vi "vision picture 1.42.vi"() -> ()   [LabVIEW 2011]
uses:
  IMAQ Image.ctl
  <vilib>/userDefined/High Color/IMAQdx.ctl
  U16 Changed__ogtk.vi
  U32 Changed__ogtk.vi
  I32 Changed__ogtk.vi
  Variant Changed__ogtk.vi
  <vilib>/vision/driver/NI_Vision_Acquisition_Software.lvlib
panel:
  in  "Zoom":sgl=1.0 min=0.1 step=0.1 format="%#_2f"
  out "Color Image":T1={"Color Image", 228380588}
  out "Image Template Out":T1
  in  "Interface Name":u16(ring) items=["Still image", "TOSHIBA Web Camera - HD", "SplitCam Video Driver", "SplitCam Video Filter", "IP Split Camera"]
  out "Paused Original Picture":picture
  out "Paused Original Image":T1={"Paused Original Image", 212497164}
  in  "Pause":bool
  in  "Play":bool
  out "Cluster Maches Color Out":T2 {"Matches Out"."Bounding Box"."y" format="%.2f"; "Matches Out"."Bounding Box"."x" format="%.2f"; "Matches Out"."Position"."y" format="%.2f"; "Matches Out"."Position"."x" format="%.2f"; "Matches Out"."Score" format="%.2f"; "Matches Out"."Scale" format="%.2f"; "Matches Out"."Angle" format="%.2f"}
  out "Cluster Shape Report Out":T3 {"Shape Report"."Score" format="%.2f"; "Shape Report"."Centroid"."y" format="%.2f"; "Shape Report"."Centroid"."x" format="%.2f"}
  out "Cluster Particle Reports (Pixels) Out":T4 {"Particle Reports (Pixels)"."Orientation" format="%.2f"; "Particle Reports (Pixels)"."Dimensions"."Height" format="%.2f"; "Particle Reports (Pixels)"."Dimensions"."Width" format="%.2f"; "Particle Reports (Pixels)"."Center of Mass"."Y" format="%.2f"; "Particle Reports (Pixels)"."Center of Mass"."X" format="%.2f"; "Particle Reports (Pixels)"."Bounding Rect"."Bottom" format="%.2f"; "Particle Reports (Pixels)"."Bounding Rect"."Right" format="%.2f"; "Particle Reports (Pixels)"."Bounding Rect"."Top" format="%.2f"; "Particle Reports (Pixels)"."Bounding Rect"."Left" format="%.2f"; "Particle Reports (Pixels)"."Number of Holes" format="%.2f"; "Particle Reports (Pixels)"."Area" format="%.2f"}
  out "Morphology Image":T1={"Morphology Image", 205500188}
  out "Threshold Image":T1={"Threshold Image", 140289436}
  out "Rect Out":T5
  out "Result Picture":picture caption="Particle Analysis"
  out "Source Image":picture
  out "Numeric Tab control":i32
  in  "Tab Control":T6(tab)
  in  "Color Mode":u16(ring) items=["RGB", "HSL", "HSV", "HSI"]
  out "Histogram":T7(graph)
  out "BCG Image":T1={"BCGLookup Image", 211850956}
  in  "Background Correction":T8={"Brightness"=128, "Contrast"=45, "Gamma"=1.0} {"Gamma" min=0.1 max=2 step=0.01 scale=0.0..2.0; "Contrast" min=1 max=90 step=1 scale=0.0..90.0; "Brightness" min=0 max=255 step=1 scale=0.0..255.0}
  in  "Subtraction":bool
  out "Backgroud In":T1
  out "Original Image":T1={"Original Image", 139855628}
  in  "Refresh":bool
  out "High Sensitivity":dbl[][](graph)
  out "Medium Sensitivity":dbl[][](graph)
  out "Color Spectrum - Low Sensitivity":dbl[][](graph)
  in  "Saturation Threshold":i32=80 min=1 max=255 step=1
  in  "Color Sensitivity":u32(ring) caption="Color Complexity" items=["Low", "Medium", "High"]
  in  "1. Threshold":bool
  in  "3. Shape":bool
  in  "Particle Connectivity Control":bool=TRUE
  in  "4. Particle Connectivity":bool
  out "MagicWand Image":T1
  in  "Shape Control":T9={"Scale Invariance"=TRUE, "Tolerance (%)"=2.0, "Connectivity"=TRUE} {"Tolerance (%)" min=0.0 max=10.0 step=0.5 format="%.2f"}
  in  "2. Morphology":bool
  in  "Morphology Control":enum32{" 1º", " 2º", " 3º", " 4º", " 5º"}(tab)
  in  "Filter":bool
  in  "Connectivity for Particle Erosion":bool=TRUE
  in  "Neighborhood":bool
  in  "Particles to Erode":i32=2
  in  "Reject Particles Touching the Image Border":bool
  in  "Connectivity for Border Rejection":bool=TRUE
  in  "Fill Holes":bool
  in  "Connectivity for Hole Filling":bool=TRUE
  in  "Morphology for Separation Erosion":bool
  in  "Separation Erosion":i32 min=0 max=20 step=1
  out "Particles":i32
  in  "Connectivity for PF":bool=TRUE
  in  "Keep/Remove PF":bool
  in  "Particle Filter Values":T11(array[cluster]) {"Measurement Parameter" items=["Center of Mass X", "Center of Mass Y", "First Pixel X", "First Pixel Y", "Bounding Rect Left", "Bounding Rect Top", "Bounding Rect Right", "Bounding Rect Bottom", "Max Feret Diameter Start X", "Max Feret Diameter Start Y", "Max Feret Diameter End X", "Max Feret Diameter End Y", "Max Horiz. Segment Length Left", "Max Horiz. Segment Length Right", "Max Horiz. Segment Length Row", "-", "Bounding Rect Width", "Bounding Rect Height", "Bounding Rect Diagonal", "Perimeter", "Convex Hull Perimeter", "Holes' Perimeter", "Max Feret Diameter", "Equivalent Ellipse Major Axis", "Equivalent Ellipse Minor Axis", "Equivalent Ellipse Minor Axis (Feret)", "Equivalent Rect Long Side", "Equivalent Rect Short Side", "Equivalent Rect Diagonal", "Equivalent Rect Short Side (Feret)", "Average Horiz. Segment Length", "Average Vert. Segment Length", "Hydraulic Radius", "Waddel Disk Diameter", "-", "Area", "Holes' Area", "Particle & Holes' Area", "Convex Hull Area", "Image Area", "-", "Number of Holes", "Number of Horiz. Segments", "Number of Vert. Segments", "-", "Orientation", "Max Feret Diameter Orientation", "-", "% Area/Image Area", "% Area/(Particle & Holes' Area)", "Ratio of Equivalent Ellipse Axes", "Ratio of Equivalent Rect Sides", "-", "Elongation Factor", "Compactness Factor", "Heywood Circularity Factor", "Type Factor", "-", "Sum X", "Sum Y", "Sum XX", "Sum XY", "Sum YY", "Sum XXX", "Sum XXY", "Sum XYY", "Sum YYY", "-", "Moment of Inertia XX", "Moment of Inertia XY", "Moment of Inertia YY", "Moment of Inertia XXX", "Moment of Inertia XXY", "Moment of Inertia XYY", "Moment of Inertia YYY", "Norm. Moment of Inertia XX", "Norm. Moment of Inertia XY", "Norm. Moment of Inertia YY", "Norm. Moment of Inertia XXX", "Norm. Moment of Inertia XXY", "Norm. Moment of Inertia XYY", "Norm. Moment of Inertia YYY", "Hu Moment 1", "Hu Moment 2", "Hu Moment 3", "Hu Moment 4", "Hu Moment 5", "Hu Moment 6", "Hu Moment 7"]; "Lower Value Range" format="%.2f"; "Upper Value Range" format="%.2f"}
  in  "Particle Filter":bool
  in  "Threshold Control":enum32{"Automatic", "Manual"}(tab)
  in  "Color Plane":i32(ring) items=["Red", "Green", "Blue", "Hue", "Saturation", "Luminance", "Value", "Intensity"]
  out "Threshold Value":i32=77
  in  "Automatic":cluster{"Object Type":u32, "Method":i32}={"Object Type"=1, "Method"=0} {"Method" items=["clustering", "entropy", "metric", "moments", "inter-class variance"]; "Object Type" items=["Bright Objects", "Dark Objects"]}
  in  "controls threshold":T12={"Threshold Color Mode"=0, "Color Value"=1, "Cluster Color"={"Histogram Red"={"Starting Value"=0.0, "Incremental Value"=1.0, "Histogram"=[0, 0, 0, 0, 0, 0, 0, 0, 0, 0, 0, 0, 0, 0, 0, 0, 0, 0, 0, 0, 0, 0, 0, 0, 0, 0, 0, 0, 0, 0, 0, 0, 0, 0, 0, 0, 0, 0, 0, 0, 1, 12, 46, 79, 116, 20, 126, 161, 147, 65, 187, 447, 707, 298, 591, 993, 827, 185, 744, 503, 189, 105, 144, 210, 115, 21, 92, 111, 97, 14, 70, 95, 76, 6, 87, 44, 60, 17, 37, 46, 30, 20, 32, 67, 21, 30, 2, 86, 20, 23, 41, 27, 36, 2, 31, 61, 16, 15, 19, 27, 24, 10, 41, 53, 15, 3, 29, 18, 25, 0, 30, 37, 28, 11, 26, 33, 9, 31, 13, 58, 9, 16, 21, 57, 11, 26, 11, 37, 13, 25, 24, 33, 16, 12, 37, 40, 5, 10, 23, 34, 24, 1, 36, 41, 18, 32, 15, 50, 13, 31, 20, 34, 42, 6, 39, 34, 23, 38, 8, 71, 16, 30, 19, 86, 30, 22, 35, 82, 50, 22, 42, 88, 45, 43, 51, 157, 113, 3, 118, 162, 157, 14, 194, 223, 65, 142, 95, 500, 488, 153, 646, 1183, 2082, 511, 3520, 4145, 4586, 1568, 3156, 2717, 1800, 238, 463, 305, 75, 29, 17, 6, 1, 0, 0, 0, 0, 0, 0, 0, 0, 0, 0, 0, 0, 0, 0, 0, 0, 0, 0, 0, 0, 0, 0, 0, 0, 0, 0, 0, 0, 0, 0, 0, 0, 0, 0, 0, 0, 0, 0, 0, 0, 0, 0, 0, 0, 0, 0, 0]}, "Histogram Blue"={"Starting Value"=0.0, "Incremental Value"=1.0, "Histogram"=[0, 0, 0, 0, 0, 0, 0, 0, 0, 0, 0, 0, 0, 0, 0, 0, 0, 0, 0, 0, 0, 0, 0, 0, 0, 0, 0, 0, 0, 0, 0, 0, 0, 0, 0, 0, 0, 0, 0, 0, 1, 12, 46, 79, 116, 20, 126, 161, 147, 65, 187, 447, 707, 298, 591, 993, 827, 185, 744, 503, 189, 105, 144, 210, 115, 21, 92, 111, 97, 14, 70, 95, 76, 6, 87, 44, 60, 17, 37, 46, 30, 20, 32, 67, 21, 30, 2, 86, 20, 23, 41, 27, 36, 2, 31, 61, 16, 15, 19, 27, 24, 10, 41, 53, 15, 3, 29, 18, 25, 0, 30, 37, 28, 11, 26, 33, 9, 31, 13, 58, 9, 16, 21, 57, 11, 26, 11, 37, 13, 25, 24, 33, 16, 12, 37, 40, 5, 10, 23, 34, 24, 1, 36, 41, 18, 32, 15, 50, 13, 31, 20, 34, 42, 6, 39, 34, 23, 38, 8, 71, 16, 30, 19, 86, 30, 22, 35, 82, 50, 22, 42, 88, 45, 43, 51, 157, 113, 3, 118, 162, 157, 14, 194, 223, 65, 142, 95, 500, 488, 153, 646, 1183, 2082, 511, 3520, 4145, 4586, 1568, 3156, 2717, 1800, 238, 463, 305, 75, 29, 17, 6, 1, 0, 0, 0, 0, 0, 0, 0, 0, 0, 0, 0, 0, 0, 0, 0, 0, 0, 0, 0, 0, 0, 0, 0, 0, 0, 0, 0, 0, 0, 0, 0, 0, 0, 0, 0, 0, 0, 0, 0, 0, 0, 0, 0, 0, 0, 0, 0]}, "Histogram Green"={"Starting Value"=0.0, "Incremental Value"=1.0, "Histogram"=[0, 0, 0, 0, 0, 0, 0, 0, 0, 0, 0, 0, 0, 0, 0, 0, 0, 0, 0, 0, 0, 0, 0, 0, 0, 0, 0, 0, 0, 0, 0, 0, 0, 0, 0, 0, 0, 0, 0, 0, 1, 12, 46, 79, 116, 20, 126, 161, 147, 65, 187, 447, 707, 298, 591, 993, 827, 185, 744, 503, 189, 105, 144, 210, 115, 21, 92, 111, 97, 14, 70, 95, 76, 6, 87, 44, 60, 17, 37, 46, 30, 20, 32, 67, 21, 30, 2, 86, 20, 23, 41, 27, 36, 2, 31, 61, 16, 15, 19, 27, 24, 10, 41, 53, 15, 3, 29, 18, 25, 0, 30, 37, 28, 11, 26, 33, 9, 31, 13, 58, 9, 16, 21, 57, 11, 26, 11, 37, 13, 25, 24, 33, 16, 12, 37, 40, 5, 10, 23, 34, 24, 1, 36, 41, 18, 32, 15, 50, 13, 31, 20, 34, 42, 6, 39, 34, 23, 38, 8, 71, 16, 30, 19, 86, 30, 22, 35, 82, 50, 22, 42, 88, 45, 43, 51, 157, 113, 3, 118, 162, 157, 14, 194, 223, 65, 142, 95, 500, 488, 153, 646, 1183, 2082, 511, 3520, 4145, 4586, 1568, 3156, 2717, 1800, 238, 463, 305, 75, 29, 17, 6, 1, 0, 0, 0, 0, 0, 0, 0, 0, 0, 0, 0, 0, 0, 0, 0, 0, 0, 0, 0, 0, 0, 0, 0, 0, 0, 0, 0, 0, 0, 0, 0, 0, 0, 0, 0, 0, 0, 0, 0, 0, 0, 0, 0, 0, 0, 0, 0]}, "Red or Hue Range"={"Minimum Value"=0.0, "Maximum Value"=155.0}, "Green or Sat Range"={"Minimum Value"=0.0, "Maximum Value"=155.0}, "Blue or Luma or Val or Inten Range"={"Minimum Value"=0.0, "Maximum Value"=155.0}}} {"Cluster Color"."Blue or Luma or Val or Inten Range" scale=0.0..255.0; "Cluster Color"."Green or Sat Range" scale=0.0..255.0; "Cluster Color"."Red or Hue Range" scale=0.0..255.0; "Threshold Color Mode" items=["RGB", "HSL", "HSV", "HSI"]}
  out "Extract Image":T1
  in  "Pen Color":u32(colorbox)=16744448
  out "Extract Picture":picture
  in  "ROI Box":T13 {"Bottom" min=0.0; "Right" min=0.0; "Top" min=0.0; "Left" min=0.0}
  in  "Search Control":T14={"Search Strategy"=0, "Color Sensitivity"=0, "Match Feature Mode"=0, "Min Score"=700.0, "# Matches"=1, "Subpixel Accuracy"=FALSE, "Min Contrast"=10, "Match Mode"=0, "Color Score Weight"=500.0, "Rotation Range (º)"=[]} {"Rotation Range (º)"."?" format="%.2f"; "Rotation Range (º)"."?" format="%.2f"; "Color Score Weight" min=0 max=1000; "Match Mode" items=["Shift Invariant", "Rotation Invariant"]; "Match Feature Mode" items=["Color and Shape", "Color", "Shape"]; "Color Sensitivity" items=["Low Sensitivity", "Medium Sensitivity", "High Sensitivity"]; "Search Strategy" items=["Conservative", "Balance", "Aggressive", "Very Aggressive"]}
  in  "Learn Control":T15={"Saturation Threshold"=80, "Ignore Black and White "=0, "Feature Mode"=0, "Ignore Color Spectra"=[], "Learn Mode"=0} {"Learn Mode" items=["All", "Shift Information", "Rotation Information"]; "Ignore Color Spectra" format="%.2f"; "Feature Mode" items=["Color and Shape", "Color", "Shape "]; "Ignore Black and White" items=["Disabled", "Ignore Black", "Ignore White", "Ignore Black and White"]; "Saturation Threshold" min=0 max=255}
  in  "Background Subtraction":bool
  in  "Learn Template":bool
  in  "Order by":u16(ring) items=["Max. Area", "Min. Area", "Max. Center of Mass", "Min. Center of Mass", ""]
  out "Color Matching":T16 {"Particle Reports (Pixels)"."Orientation" format="%.2f"; "Particle Reports (Pixels)"."Dimensions"."Height" format="%.2f"; "Particle Reports (Pixels)"."Dimensions"."Width" format="%.2f"; "Particle Reports (Pixels)"."Center of Mass"."Y" format="%.2f"; "Particle Reports (Pixels)"."Center of Mass"."X" format="%.2f"; "Particle Reports (Pixels)"."Bounding Rect"."Bottom" format="%.2f"; "Particle Reports (Pixels)"."Bounding Rect"."Right" format="%.2f"; "Particle Reports (Pixels)"."Bounding Rect"."Top" format="%.2f"; "Particle Reports (Pixels)"."Bounding Rect"."Left" format="%.2f"; "Particle Reports (Pixels)"."Number of Holes" format="%.2f"; "Particle Reports (Pixels)"."Area" format="%.2f"}
  out "Color Matching":T17 {"Matches Out"."Bounding Box"."y" format="%.2f"; "Matches Out"."Bounding Box"."x" format="%.2f"; "Matches Out"."Position"."y" format="%.2f"; "Matches Out"."Position"."x" format="%.2f"; "Matches Out"."Score" format="%.2f"; "Matches Out"."Scale" format="%.2f"; "Matches Out"."Angle" format="%.2f"}
  in  "Order by":u16(ring) items=["Max. Score", "Min. Score", "Max. Position", "Min. Position"]
  in  "Show Results":u16(slide)
  out "Global Result":T18 {"Variance"."Ey2" format="%.2f"; "Variance"."Ex2" format="%.2f"; "Standard Deviation"."Ey" format="%.2f"; "Standard Deviation"."Ex" format="%.2f"; "Position"."Y" format="%.2f"; "Position"."X" format="%.2f"}
  in  "Order by":u16(ring) items=["Max. Object Size", "Min. Object Size", "Max. Score", "Min. Score"]
  out "Particle Analysis":T19 {"Shape Report"."Score" format="%.2f"; "Shape Report"."Centroid"."y" format="%.2f"; "Shape Report"."Centroid"."x" format="%.2f"}
  in  "Show Draw Point":T20={"Show Text"=TRUE, "Show Center"=TRUE, "Show Bounding Box"=TRUE, "Show Angle"=FALSE}
  out "stop 2":bool
  out "Acquiring":bool
  in  "stop":bool
  # "Color Histogram"
  # "Color Spectrum"
  # "Controls"
  # "If the automatic threshold does not work, try manual mode. Clear any particle with the morphology control. Click any shape to find."
  # "R/H"
  # "G/S"
  # "B/LVI"
  # "ROI"
  # "Select an object taking a square area about it on the output image. Modify the color of the ROI bounding box as desired"
  # "1. Choose the learning mode before the capturing process if wanted"
  # "2. Once learn, the searching process can be optimized"
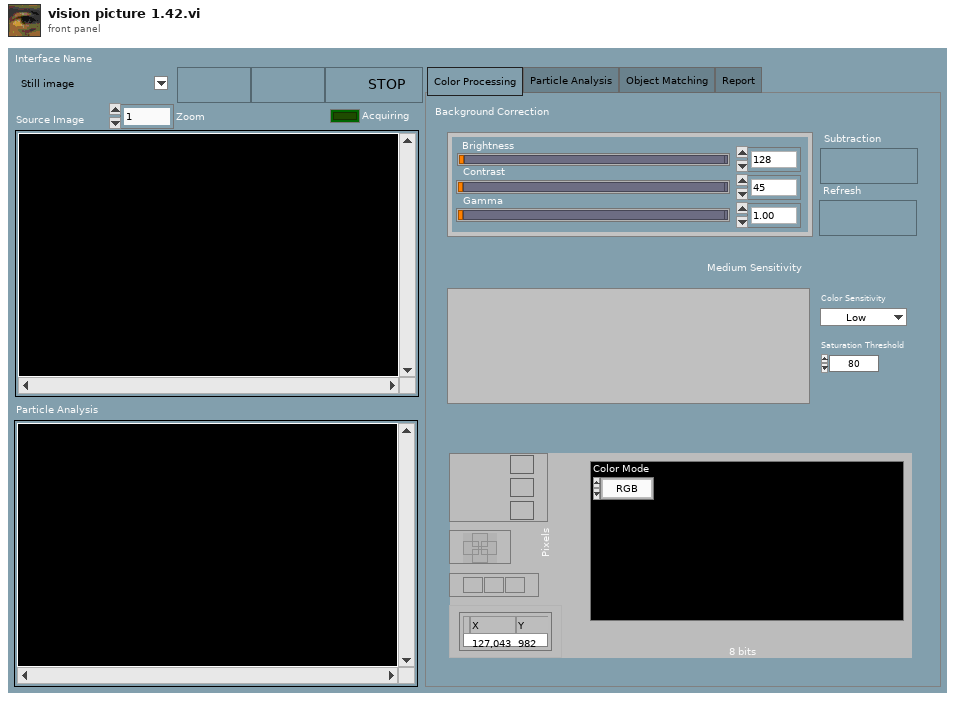
[diagram p1: front panel]
types:
  T1 = typedef "IMAQ Image.ctl" = cluster{string, u32}
  T2 = cluster{"Matches Out":cluster{"Position":cluster{"x":sgl, "y":sgl}, "Angle":sgl, "Scale":sgl, "Score":sgl, "Bounding Box":cluster{"x":sgl, "y":sgl}[]}[], "N. Matches Color":i32}
  T3 = cluster{"Shape Report":cluster{"Global Rectangle":cluster{"x1Left":i32, "y1Top":i32, "x2Right":i32, "y2Bottom":i32}, "Centroid":cluster{"x":sgl, "y":sgl}, "Object Size":u32, "Score":dbl}[], "N. Matches Shape":i32}
  T4 = cluster{"Particle Reports (Pixels)":cluster{"Area":dbl, "Number of Holes":dbl, "Bounding Rect":cluster{"Left":dbl, "Top":dbl, "Right":dbl, "Bottom":dbl}, "Center of Mass":cluster{"X":dbl, "Y":dbl}, "Orientation":dbl, "Dimensions":cluster{"Width":dbl, "Height":dbl}}[], "N. Particles Report":i32}
  T5 = cluster{"Left":i32, "Top":i32, "Right":i32, "Bottom":i32}
  T6 = enum32{"Color Processing", "Particle Analysis", "Object Matching", "Report"}
  T7 = cluster{"Starting Value":sgl, "Incremental Value":sgl, "Histogram":u32[]}[]
  T8 = cluster{"Brightness":i32, "Contrast":i32, "Gamma":sgl}
  T9 = cluster{"Scale Invariance":bool, "Tolerance (%)":dbl, "Connectivity":bool}
  T10 = typedef "Particle Parameters" = i32
  T11 = cluster{"Measurement Parameter":T10, "Lower Value Range":dbl, "Upper Value Range":dbl, "Range":bool, "Measurement Type":bool}[]
  T12 = cluster{"Threshold Color Mode":u16, "Color Value":i32, "Cluster Color":cluster{"Histogram Red":cluster{"Starting Value":sgl, "Incremental Value":sgl, "Histogram":u32[]}, "Histogram Blue":cluster{"Starting Value":sgl, "Incremental Value":sgl, "Histogram":u32[]}, "Histogram Green":cluster{"Starting Value":sgl, "Incremental Value":sgl, "Histogram":u32[]}, "Red or Hue Range":cluster{"Minimum Value":sgl, "Maximum Value":sgl}, "Green or Sat Range":cluster{"Minimum Value":sgl, "Maximum Value":sgl}, "Blue or Luma or Val or Inten Range":cluster{"Minimum Value":sgl, "Maximum Value":sgl}}}
  T13 = cluster{"Left":dbl, "Top":dbl, "Right":dbl, "Bottom":dbl}
  T14 = cluster{"Search Strategy":u32, "Color Sensitivity":u32, "Match Feature Mode":u32, "Min Score":sgl, "# Matches":i32, "Subpixel Accuracy":bool, "Min Contrast":i32, "Match Mode":u16, "Color Score Weight":sgl, "Rotation Range (º)":cluster{sgl, sgl}[]}
  T15 = cluster{"Saturation Threshold":i32, "Ignore Black and White ":u32, "Feature Mode":u32, "Ignore Color Spectra":dbl[][], "Learn Mode":u16}
  T16 = cluster{"Particle Reports (Pixels)":cluster{"Area":dbl, "Number of Holes":dbl, "Bounding Rect":cluster{"Left":dbl, "Top":dbl, "Right":dbl, "Bottom":dbl}, "Center of Mass":cluster{"X":dbl, "Y":dbl}, "Orientation":dbl, "Dimensions":cluster{"Width":dbl, "Height":dbl}}[], "Total Matches":i32}
  T17 = cluster{"Matches Out":cluster{"Position":cluster{"x":sgl, "y":sgl}, "Angle":sgl, "Scale":sgl, "Score":sgl, "Bounding Box":cluster{"x":sgl, "y":sgl}[]}[], "Total Matches":i32}
  T18 = cluster{"Position":cluster{"X":sgl, "Y":sgl}, "Standard Deviation":cluster{"Ex":sgl, "Ey":sgl}, "Variance":cluster{"Ex2":sgl, "Ey2":sgl}, "Object Size":u32}
  T19 = cluster{"Shape Report":cluster{"Global Rectangle":cluster{"x1Left":i32, "y1Top":i32, "x2Right":i32, "y2Bottom":i32}, "Centroid":cluster{"x":sgl, "y":sgl}, "Object Size":u32, "Score":dbl}[], "Total Matches":i32}
  T20 = cluster{"Show Text":bool, "Show Center":bool, "Show Bounding Box":bool, "Show Angle":bool}
  T21 = typedef "IMAQdx.ctl" = refnum<k21>
  T22 = cluster{"[0]":i32, "[0]":i32, "[1]":i32, "[1]":i32}
  T23 = cluster{"Position":cluster{"x":sgl, "y":sgl}, "Angle":sgl, "Scale":sgl, "Score":sgl, "Bounding Box":cluster{"x":sgl, "y":sgl}[]}
  T24 = cluster{"Type":u32, "Version":u32, "Flags":u32, "SerialNumberHigh":u32, "SerialNumberLow":u32, "BusType":u32, "InterfaceName":string, "VendorName":string, "ModelName":string, "CameraFileName":string, "CameraAttributeURL":string}[]
  T25 = cluster{"Type":u32, "Version":u32, "Flags":u32, "SerialNumberHigh":u32, "SerialNumberLow":u32, "BusType":u32, "InterfaceName":string, "VendorName":string, "ModelName":string, "CameraFileName":string, "CameraAttributeURL":string}
  T26 = typedef "Image Type" = u32
  T27 = typedef "imagedata.ctl" = cluster{"image type":i32, "image depth":i32, "image":u8[], "mask":u8[], "colors":u32[], "Rectangle":cluster{"left":i16, "top":i16, "right":i16, "bottom":i16}}
  T28 = cluster{"Position":cluster{"x":sgl, "y":sgl}, "Angle":sgl, "Scale":sgl, "Score":sgl, "Bounding Box":cluster{"x":sgl, "y":sgl}[]}[]
  T29 = cluster{"Area":dbl, "Number of Holes":dbl, "Bounding Rect":cluster{"Left":dbl, "Top":dbl, "Right":dbl, "Bottom":dbl}, "Center of Mass":cluster{"X":dbl, "Y":dbl}, "Orientation":dbl, "Dimensions":cluster{"Width":dbl, "Height":dbl}}[]
  T30 = cluster{"Global Rectangle":cluster{"x1Left":i32, "y1Top":i32, "x2Right":i32, "y2Bottom":i32}, "Centroid":cluster{"x":sgl, "y":sgl}, "Object Size":u32, "Score":dbl}[]
  T31 = cluster{"Shape Report 2":cluster{"Global Rectangle":cluster{"x1Left":i32, "y1Top":i32, "x2Right":i32, "y2Bottom":i32}, "Centroid":cluster{"x":sgl, "y":sgl}, "Object Size":u32, "Score":dbl}[], "N. Matches Shape":i32}
  T32 = cluster{"Particle Reports (Pixels) 2":cluster{"Area":dbl, "Number of Holes":dbl, "Bounding Rect":cluster{"Left":dbl, "Top":dbl, "Right":dbl, "Bottom":dbl}, "Center of Mass":cluster{"X":dbl, "Y":dbl}, "Orientation":dbl, "Dimensions":cluster{"Width":dbl, "Height":dbl}}[], "N. Particles Report":i32}
  T33 = cluster{"Position":cluster{"X":sgl, "Y":sgl}, "Standar Desviation":cluster{"Ex":sgl, "Ey":sgl}, "Variance":cluster{"Ex2":sgl, "Ey2":sgl}, "Object Size":u32}
  T34 = typedef "LVMouseTypeDef.ctl" = cluster{"Mouse Position":cluster{"X":i32, "Y":i32}, "Mouse Modifiers":cluster{"Button Down":bool, "Shift Mod":bool, "Menu Mod":bool, "Option Mod":bool}}
  T35 = typedef "Vision Info Type" = u32
  T36 = cluster{"Matches Out":cluster{"Position":cluster{"x":sgl, "y":sgl}, "Angle":sgl, "Scale":sgl, "Score":sgl, "Bounding Box":cluster{"x":sgl, "y":sgl}[]}[], "Number of Matches Out":i32}
  T37 = cluster{"[0]":bool, "[0]":bool, "[1]":bool, "[1]":bool}
  T38 = cluster{"Starting Value":sgl, "Incremental Value":sgl, "Histogram":u32[]}
  T39 = cluster{"Histogram Red":cluster{"Starting Value":sgl, "Incremental Value":sgl, "Histogram":u32[]}, "Histogram Blue":cluster{"Starting Value":sgl, "Incremental Value":sgl, "Histogram":u32[]}, "Histogram Green":cluster{"Starting Value":sgl, "Incremental Value":sgl, "Histogram":u32[]}, "Red or Hue Range":cluster{"Minimum Value":sgl, "Maximum Value":sgl}, "Green or Sat Range":cluster{"Minimum Value":sgl, "Maximum Value":sgl}, "Blue or Luma or Val or Inten Range":cluster{"Minimum Value":sgl, "Maximum Value":sgl}}
  T40 = cluster{"Minimum Value":sgl, "Maximum Value":sgl}
  T41 = cluster{"Particle Reports (Pixels)":cluster{"Area":dbl, "Number of Holes":dbl, "Bounding Rect":cluster{"Left":dbl, "Top":dbl, "Right":dbl, "Bottom":dbl}, "Center of Mass":cluster{"X":dbl, "Y":dbl}, "Orientation":dbl, "Dimensions":cluster{"Width":dbl, "Height":dbl}}[], "Number of Particles":i32}
  T42 = cluster{"Button Down":bool, "Shift Mod":bool, "Menu Mod":bool, "Option Mod":bool}
  T43 = cluster{"Shape Report":cluster{"Global Rectangle":cluster{"x1Left":i32, "y1Top":i32, "x2Right":i32, "y2Bottom":i32}, "Centroid":cluster{"x":sgl, "y":sgl}, "Object Size":u32, "Score":dbl}[], "Number of Matches":i32}
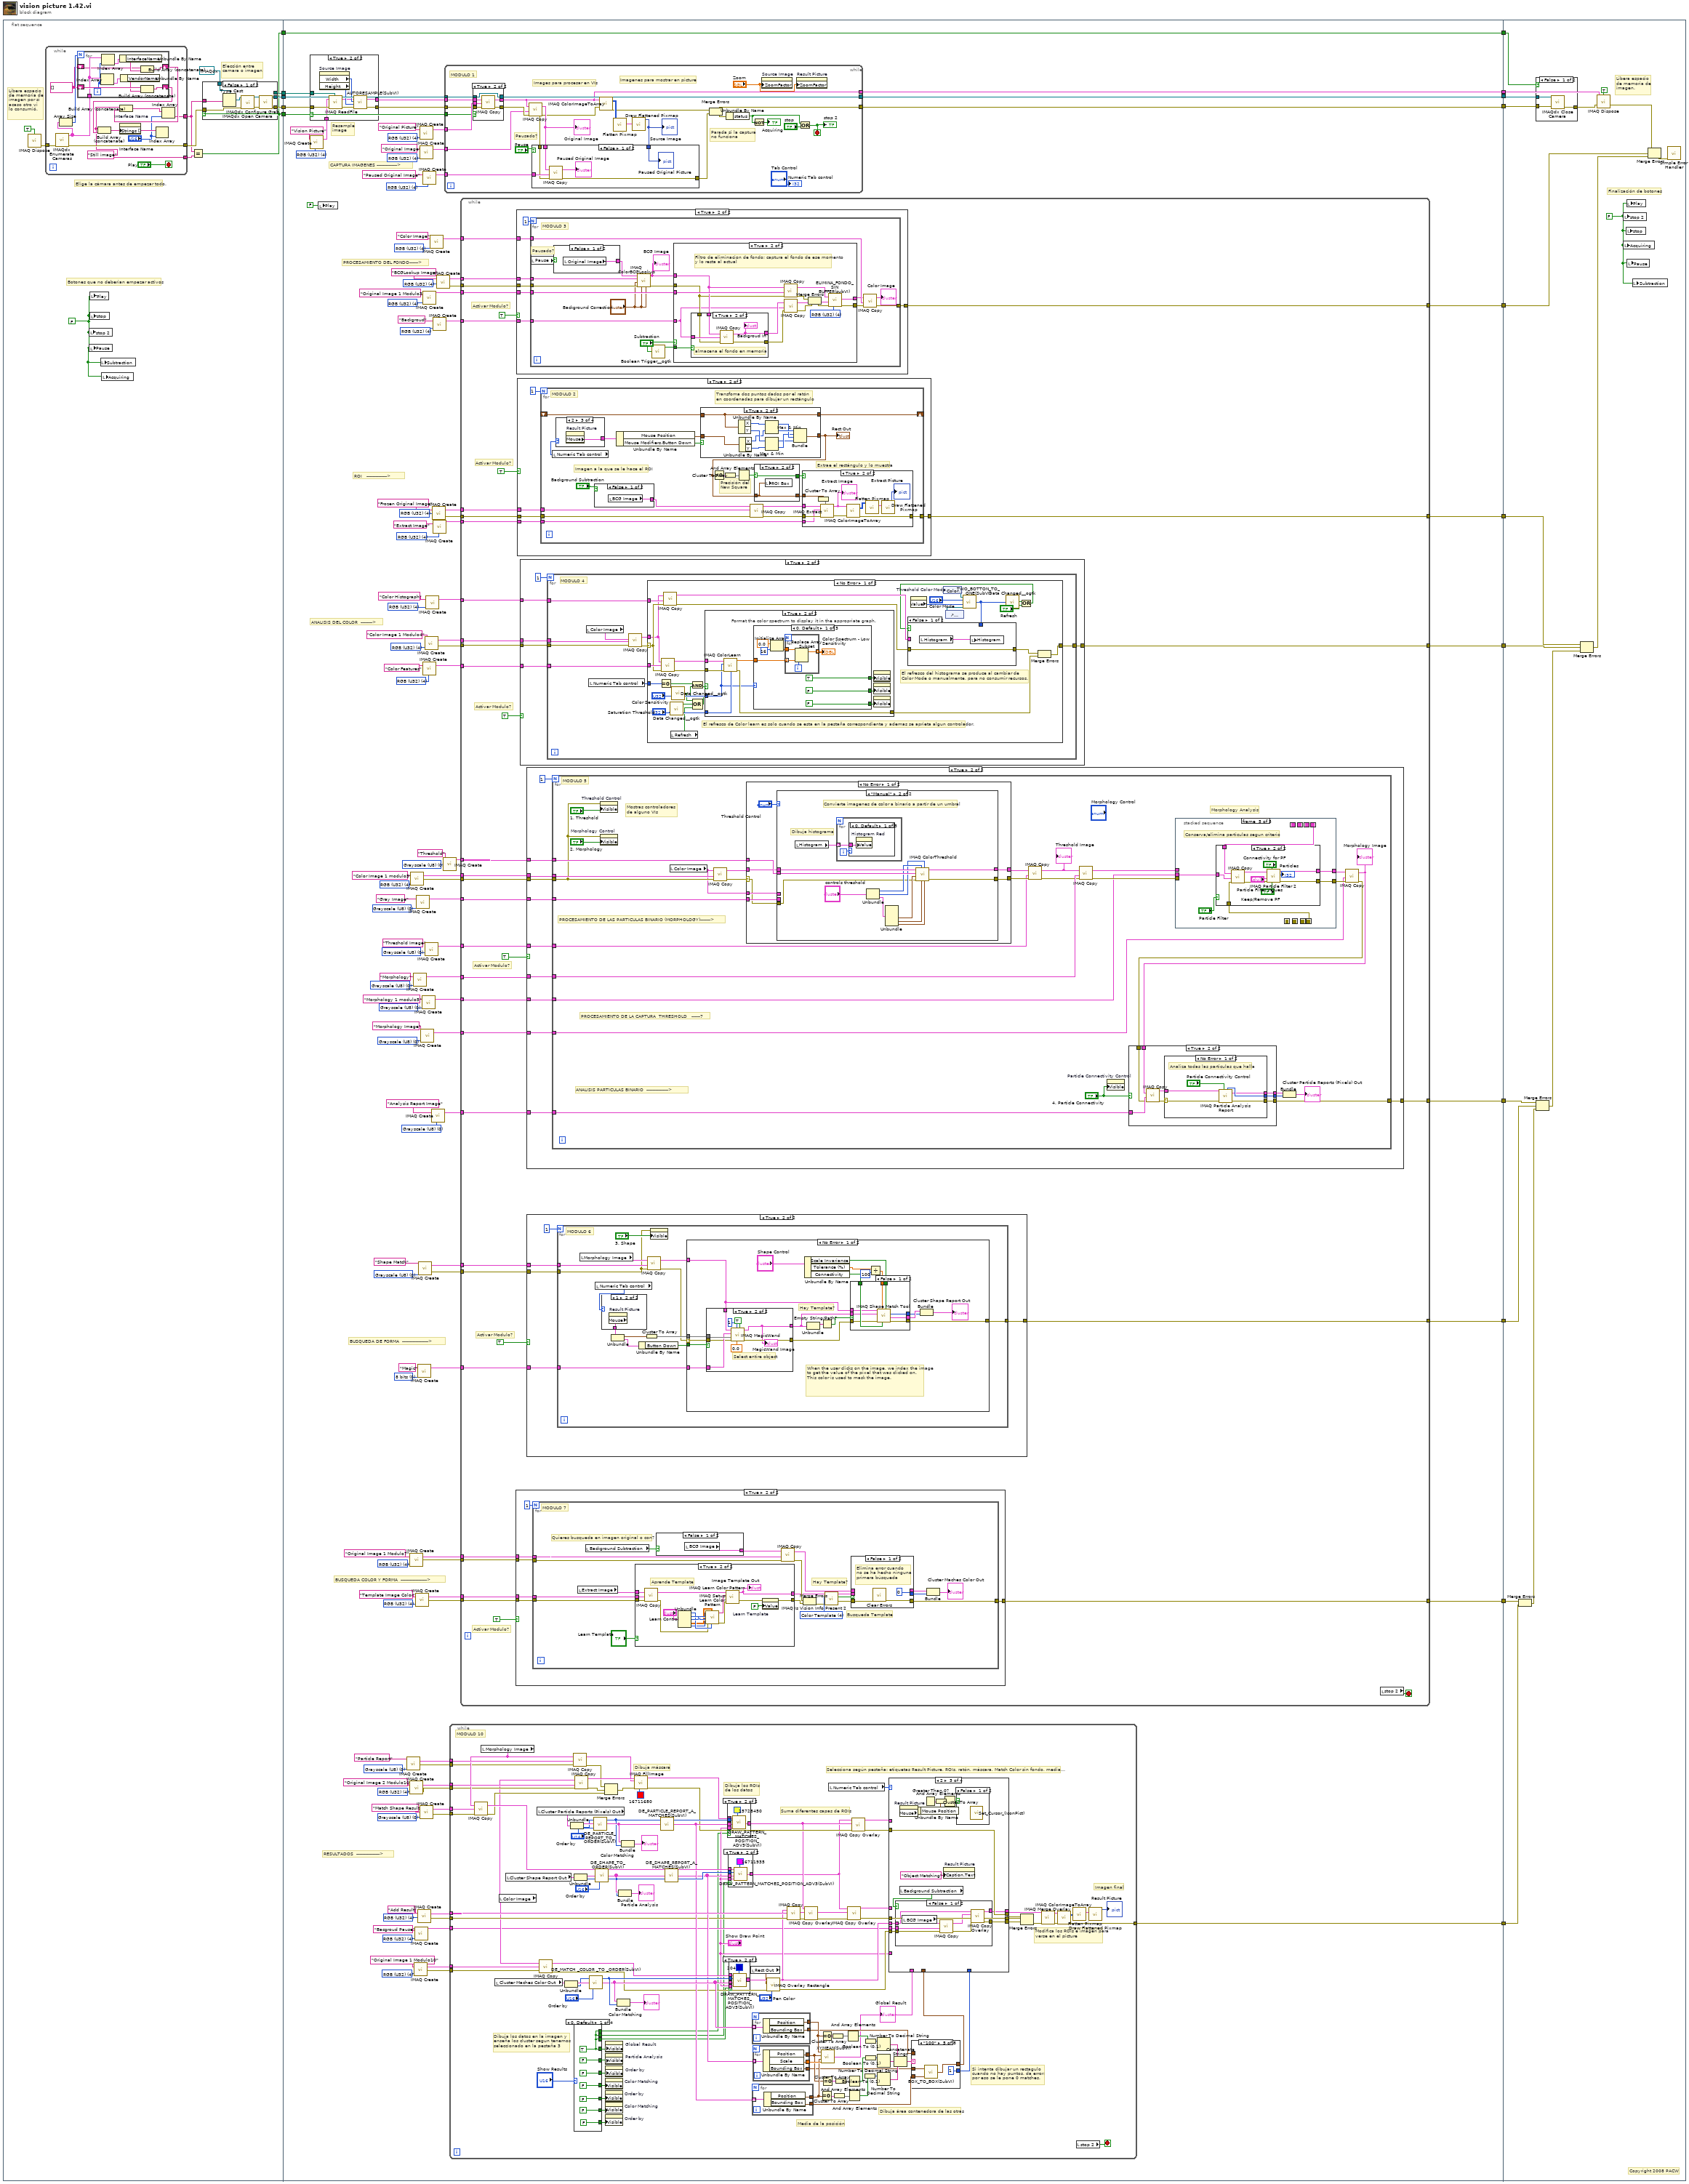
[diagram p0: block diagram]
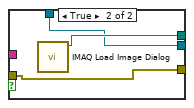
[diagram p2: hidden frame]
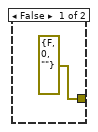
[diagram p4: hidden frame]
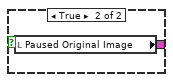
[diagram p5: hidden frame]
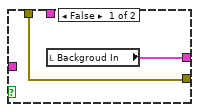
[diagram p7: hidden frame]
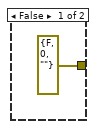
[diagram p8: hidden frame]
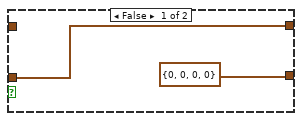
[diagram p9: hidden frame]
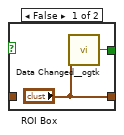
[diagram p10: hidden frame]
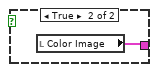
[diagram p11: hidden frame]
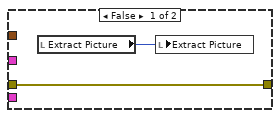
[diagram p15: hidden frame]
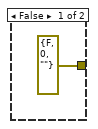
[diagram p16: hidden frame]
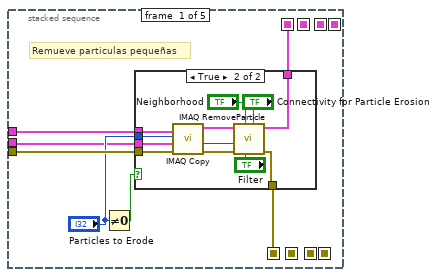
[diagram p19: hidden frame]
diagram:
  n1 = flat-sequence {
    tunnel: [w20] -> w16
    tunnel: [w17] -> w5
    tunnel: [w21] -> w4
    tunnel: [w22] -> w3
    tunnel: [w17] -> w2
    tunnel: w16 -> [w184]
    tunnel: [w178] -> w15
    tunnel: [w183] -> w14
    tunnel: [w177] -> w13
    tunnel: [w182] -> w12
    tunnel: [w180] -> w11
    tunnel: [w181] -> w10
    tunnel: [w179] -> w9
    tunnel: [w95] -> w8
    tunnel: [w94] -> w7
    tunnel: [w83] -> w6
    tunnel: w5 -> [w70]
    tunnel: w4 -> [w65]
    tunnel: w3 -> [w72]
    tunnel: w2 -> [w62]
    tunnel: [w62] -> w1
    tunnel: w15 -> [w1089]
    tunnel: w14 -> [w1087]
    tunnel: w13 -> [w1091]
    tunnel: w12 -> [w1101]
    tunnel: w11 -> [w1094]
    tunnel: w10 -> [w1093]
    tunnel: w9 -> [w1098]
    tunnel: w8 -> [w1095]
    tunnel: w7 -> [w1096]
    tunnel: w6 -> [w1090]
    tunnel: w1 -> [w1086]
    frame #0 {
      w18 = FALSE
      # "Libera espacio\nde memoria de\nimagen por si\nacaso otro vi\nlo consumió."
      # "Elección entre camara o imagen"
      # "Elige la cámara antes de empezar todo."
      # "Botones que no deberian empezar activos"
      n2 = call "IMAQ Dispose"("All Images? (No)"=TRUE) -> ("error out"=w24:errorcluster)  [unwired: 2 in, 3 out]
      n3 = while {
        tunnel: [w40] -> w25
        tunnel: w24 -> [w51]
        tunnel: [w42] -> w26
        tunnel: [w50] -> w27
        stop <- "Play" stop-if-true
        w44 = string[] []
        w42 = "Still image"
        n4 = call <vilib>:"IMAQdx Enumerate Cameras.vi"("error in"=w51) -> ("error out"=w50:errorcluster, "Camera Information Array"=w48:T24)  [unwired: 9 in]
        n5 = Array Size(array=w48) -> (size(s)=w45:i32)
        n6 = for {
          N: w45 -> [_]
          tunnel: w48 -> [w54]
          shift-right: [w60] -> w46
          shift-left: w44 -> [w59]
          shift-right: [w55] -> w41
          shift-left: w44 -> [w53]
          i -> [w52]
          n7 = Index Array(array=w54, index=w52) -> (element=w61:T25)
          n8 = Index Array(array=w54, index=w52) -> (element=w57:T25)
          n9 = Unbundle By Name(w57) -> ("InterfaceName"=w56:string)
          n10 = Unbundle By Name(w61) -> ("VendorName"=w58:string)
          n11 = Build Array (concatenate)(w59, w58) -> (w60:string[])
          n12 = Build Array (concatenate)(w53, w56) -> (w55:string[])
        }
        n13 = Build Array (concatenate)(w42, w46) -> (w47:string[])
        n14 = property on="Interface Name" class="Ring (strict)"("Strings []"=w47) -> ()  [unwired: 2 in, 2 out]
        n15 = Build Array (concatenate)(w42, w41) -> (w43:string[])
        n16 = Index Array(array=w47, index="Interface Name") -> ()  [unwired: 1 out]
        n17 = Index Array(array=w43, index="Interface Name") -> (element=w40:string)
      }
      n18 = local write "stop 2"(w18) -> ()
      n19 = local write "Pause"(w18) -> ()
      n20 = local write "Play"(w18) -> ()
      n21 = local write "stop"(w18) -> ()
      n22 = local write "Subtraction"(w18) -> ()
      n23 = local write "Acquiring"(w18) -> ()
      n24 = Equal?(x=w25, y=w26) -> (x = y?=w17:bool)
      n25 = case shown="False" w17 {
        tunnel: [w32 w37] -> w22
        tunnel: w25 -> [w31 _]
        tunnel: [_ w38] -> w21
        tunnel: w27 -> [w33 w37]
        tunnel: [w29 w36] -> w20
        tunnel: T21 refnum ("Session In") -> [w28 w36]
        frame False {
          n26 = Type Cast(type=w28, x=w31) -> (*(type *) &x=w30:T21)
          n27 = call <vilib>:"IMAQdx Open Camera.vi"("error in"=w33, "Session In"=w30) -> ("error out"=w34:errorcluster, "Session Out"=w35:T21)  [unwired: 8 in]
          n28 = call <vilib>:"IMAQdx Configure Grab.vi"("error in"=w34, "Session In"=w35) -> ("error out"=w32:errorcluster, "Session Out"=w29:T21)  [unwired: 8 in]
        }
        frame True {
          n29 = call "IMAQ Load Image Dialog"() -> ("Path"=w38:path)  [unwired: 7 in, 4 out]
        }
      }
    }
    frame #1 {
      w67 = T26 4 items=["Grayscale (U8)", "Grayscale (I16)", "Grayscale (SGL)", "Complex (CSG)", "RGB (U32)", "HSL (U32)", "RGB (U64)"] ("Image Type")
      w76 = T26 4 items=["Grayscale (U8)", "Grayscale (I16)", "Grayscale (SGL)", "Complex (CSG)", "RGB (U32)", "HSL (U32)", "RGB (U64)"] ("Image Type")
      w79 = T26 4 items=["Grayscale (U8)", "Grayscale (I16)", "Grayscale (SGL)", "Complex (CSG)", "RGB (U32)", "HSL (U32)", "RGB (U64)"] ("Image Type")
      w82 = T26 4 items=["Grayscale (U8)", "Grayscale (I16)", "Grayscale (SGL)", "Complex (CSG)", "RGB (U32)", "HSL (U32)", "RGB (U64)"] ("Image Type")
      w85 = T26 4 items=["Grayscale (U8)", "Grayscale (I16)", "Grayscale (SGL)", "Complex (CSG)", "RGB (U32)", "HSL (U32)", "RGB (U64)"] ("Image Type")
      w89 = T26 4 items=["Grayscale (U8)", "Grayscale (I16)", "Grayscale (SGL)", "Complex (CSG)", "RGB (U32)", "HSL (U32)", "RGB (U64)"] ("Image Type")
      w92 = T26 4 items=["Grayscale (U8)", "Grayscale (I16)", "Grayscale (SGL)", "Complex (CSG)", "RGB (U32)", "HSL (U32)", "RGB (U64)"] ("Image Type")
      w99 = T26 4 items=["Grayscale (U8)", "Grayscale (I16)", "Grayscale (SGL)", "Complex (CSG)", "RGB (U32)", "HSL (U32)", "RGB (U64)"] ("Image Type")
      w102 = T26 4 items=["Grayscale (U8)", "Grayscale (I16)", "Grayscale (SGL)", "Complex (CSG)", "RGB (U32)", "HSL (U32)", "RGB (U64)"] ("Image Type")
      w109 = T26 4 items=["Grayscale (U8)", "Grayscale (I16)", "Grayscale (SGL)", "Complex (CSG)", "RGB (U32)", "HSL (U32)", "RGB (U64)"] ("Image Type")
      w111 = T26 4 items=["Grayscale (U8)", "Grayscale (I16)", "Grayscale (SGL)", "Complex (CSG)", "RGB (U32)", "HSL (U32)", "RGB (U64)"] ("Image Type")
      w117 = T26 0 items=["Grayscale (U8)", "Grayscale (I16)", "Grayscale (SGL)", "Complex (CSG)", "RGB (U32)", "HSL (U32)", "RGB (U64)"] ("Image Type")
      w64 = u32 0 items=["8 bits", "16 bits", "Float", "Complex", "RGB", "HSL"] ("Image Type")
      w116 = T26 0 items=["Grayscale (U8)", "Grayscale (I16)", "Grayscale (SGL)", "Complex (CSG)", "RGB (U32)", "HSL (U32)", "RGB (U64)"] ("Image Type")
      w137 = T26 0 items=["Grayscale (U8)", "Grayscale (I16)", "Grayscale (SGL)", "Complex (CSG)", "RGB (U32)", "HSL (U32)", "RGB (U64)"] ("Image Type")
      w139 = T26 0 items=["Grayscale (U8)", "Grayscale (I16)", "Grayscale (SGL)", "Complex (CSG)", "RGB (U32)", "HSL (U32)", "RGB (U64)"] ("Image Type")
      w141 = T26 0 items=["Grayscale (U8)", "Grayscale (I16)", "Grayscale (SGL)", "Complex (CSG)", "RGB (U32)", "HSL (U32)", "RGB (U64)"] ("Image Type")
      w135 = T26 0 items=["Grayscale (U8)", "Grayscale (I16)", "Grayscale (SGL)", "Complex (CSG)", "RGB (U32)", "HSL (U32)", "RGB (U64)"] ("Image Type")
      w130 = T26 0 items=["Grayscale (U8)", "Grayscale (I16)", "Grayscale (SGL)", "Complex (CSG)", "RGB (U32)", "HSL (U32)", "RGB (U64)"] ("Image Type")
      w131 = T26 0 items=["Grayscale (U8)", "Grayscale (I16)", "Grayscale (SGL)", "Complex (CSG)", "RGB (U32)", "HSL (U32)", "RGB (U64)"] ("Image Type")
      w133 = T26 4 items=["Grayscale (U8)", "Grayscale (I16)", "Grayscale (SGL)", "Complex (CSG)", "RGB (U32)", "HSL (U32)", "RGB (U64)"] ("Image Type")
      w151 = T26 4 items=["Grayscale (U8)", "Grayscale (I16)", "Grayscale (SGL)", "Complex (CSG)", "RGB (U32)", "HSL (U32)", "RGB (U64)"] ("Image Type")
      w149 = T26 4 items=["Grayscale (U8)", "Grayscale (I16)", "Grayscale (SGL)", "Complex (CSG)", "RGB (U32)", "HSL (U32)", "RGB (U64)"] ("Image Type")
      w147 = T26 4 items=["Grayscale (U8)", "Grayscale (I16)", "Grayscale (SGL)", "Complex (CSG)", "RGB (U32)", "HSL (U32)", "RGB (U64)"] ("Image Type")
      w154 = T26 4 items=["Grayscale (U8)", "Grayscale (I16)", "Grayscale (SGL)", "Complex (CSG)", "RGB (U32)", "HSL (U32)", "RGB (U64)"] ("Image Type")
      w164 = T26 0 items=["Grayscale (U8)", "Grayscale (I16)", "Grayscale (SGL)", "Complex (CSG)", "RGB (U32)", "HSL (U32)", "RGB (U64)"] ("Image Type")
      w167 = T26 4 items=["Grayscale (U8)", "Grayscale (I16)", "Grayscale (SGL)", "Complex (CSG)", "RGB (U32)", "HSL (U32)", "RGB (U64)"] ("Image Type")
      w169 = T26 0 items=["Grayscale (U8)", "Grayscale (I16)", "Grayscale (SGL)", "Complex (CSG)", "RGB (U32)", "HSL (U32)", "RGB (U64)"] ("Image Type")
      w171 = T26 4 items=["Grayscale (U8)", "Grayscale (I16)", "Grayscale (SGL)", "Complex (CSG)", "RGB (U32)", "HSL (U32)", "RGB (U64)"] ("Image Type")
      w173 = T26 4 items=["Grayscale (U8)", "Grayscale (I16)", "Grayscale (SGL)", "Complex (CSG)", "RGB (U32)", "HSL (U32)", "RGB (U64)"] ("Image Type")
      w176 = T26 4 items=["Grayscale (U8)", "Grayscale (I16)", "Grayscale (SGL)", "Complex (CSG)", "RGB (U32)", "HSL (U32)", "RGB (U64)"] ("Image Type")
      # "Resample\nimage"
      # "BUSQUEDA DE FORMA  ------------------>"
      # "BUSQUEDA COLOR Y FORMA  ------------------>"
      # "ANALISIS DEL COLOR  -------->"
      # "PROCESAMIENTO DEL FONDO------>"
      # "ROI   -------------->"
      # "RESULTADOS  ---------------->"
      # "CAPTURA IMAGENES -------------->"
      n30 = call "IMAQ Create.vi"("Image Name"="Vision Picture", "Image Type"=w67) -> ("New Image"=w66:T1)  [unwired: 2 in, 2 out]
      n31 = case shown="True" w70 {
        tunnel: w72 -> [w186 w191]
        tunnel: [w186 w190] -> w71
        tunnel: [w185 w189] -> w69
        tunnel: w66 -> [w185 w188]
        tunnel: w65 -> [_ w187]
        frame False {
        }
        frame True {
          n32 = property on="Source Image" class="Pict"() -> ("Width"=w195:u32, "Height"=w194:u32)  [unwired: 2 in, 2 out]
          n33 = call "IMAQ ReadFile"("File Path"=w187, "error in (no error)"=w191, "Image"=w188) -> ("error out"=w192:errorcluster, "Image Out"=w193:T1)  [unwired: 2 in, 5 out]
          n34 = call "AUTORESAMPLE(SubVI).vi"("Error In"=w192, "Y Resolution"=w194, "X Resolution"=w195, "Image In"=w193) -> ("Error Out"=w190:errorcluster, "Image Resize Out"=w189:T1)  [unwired: 4 in, 2 out]
        }
      }
      n35 = local write "Play"(FALSE) -> ()
      n36 = call "IMAQ Create.vi"("Image Name"="Particle Report", "Image Type"=w169) -> ("New Image"=w163:T1, "error out"=w162:errorcluster)  [unwired: 2 in, 1 out]
      n37 = call "IMAQ Create.vi"("Image Name"="Original Image 1 Modulo7", "Image Type"=w109) -> ("New Image"=w107:T1, "error out"=w106:errorcluster)  [unwired: 2 in, 1 out]
      n38 = call "IMAQ Create.vi"("Image Name"="Original Image 2 Modulo10", "Image Type"=w167) -> ("New Image"=w161:T1, "error out"=w160:errorcluster)  [unwired: 2 in, 1 out]
      n39 = call "IMAQ Create.vi"("Image Name"="Color Image 1 modulo5", "Image Type"=w133) -> ("New Image"=w121:T1, "error out"=w122:errorcluster)  [unwired: 2 in, 1 out]
      n40 = call "IMAQ Create.vi"("Image Name"="Morphology", "Image Type"=w141) -> ("New Image"=w125:T1)  [unwired: 2 in, 2 out]
      n41 = call "IMAQ Create.vi"("Image Name"="Original Image 1 Modulo10", "Image Type"=w171) -> ("New Image"=w156:T1, "error out"=w155:errorcluster)  [unwired: 2 in, 1 out]
      n42 = call "IMAQ Create.vi"("Image Name"="Bacgroud Pause", "Image Type"=w79) -> ("New Image"=w77:T1)  [unwired: 2 in, 2 out]
      n43 = call "IMAQ Create.vi"("Image Name"="Template Image Color", "Image Type"=w111) -> ("New Image"=w105:T1, "error out"=w104:errorcluster)  [unwired: 2 in, 1 out]
      n44 = call "IMAQ Create.vi"("Image Name"="Gray Image", "Image Type"=w130) -> ("New Image"=w123:T1)  [unwired: 2 in, 2 out]
      n45 = call "IMAQ Create.vi"("Image Name"="Add Result", "Image Type"=w173) -> ("New Image"=w157:T1, "error out"=w93:errorcluster)  [unwired: 2 in, 1 out]
      n46 = call "IMAQ Create.vi"("Image Name"="Magic", "Image Type"=w64) -> ("New Image"=w115:T1)  [unwired: 2 in, 2 out]
      n47 = call "IMAQ Create.vi"("Image Name"="Shape Match", "Image Type"=w117) -> ("New Image"=w114:T1, "error out"=w113:errorcluster)  [unwired: 2 in, 1 out]
      n48 = call "IMAQ Create.vi"("Image Name"="Original Picture", "Image Type"=w176) -> ("New Image"=w174:T1)  [unwired: 2 in, 2 out]
      n49 = call "IMAQ Create.vi"("Image Name"="Original Image", "Image Type"=w102) -> ("New Image"=w100:T1)  [unwired: 2 in, 2 out]
      n50 = call "IMAQ Create.vi"("Image Name"="Match Shape Result", "Image Type"=w164) -> ("New Image"=w159:T1, "error out"=w158:errorcluster)  [unwired: 2 in, 1 out]
      n51 = call "IMAQ Create.vi"("Image Name"="Morphology Image", "Image Type"=w139) -> ("New Image"=w127:T1)  [unwired: 2 in, 2 out]
      n52 = call "IMAQ Create.vi"("Image Name"="Morphology 1 modulo5", "Image Type"=w137) -> ("New Image"=w126:T1)  [unwired: 2 in, 2 out]
      n53 = call "IMAQ Create.vi"("Image Name"="Paused Original Image", "Image Type"=w82) -> ("New Image"=w80:T1)  [unwired: 2 in, 2 out]
      n54 = call "IMAQ Create.vi"("Image Name"="Original Image 1 Modulo3", "Image Type"=w89) -> ("New Image"=w87:T1)  [unwired: 2 in, 2 out]
      n55 = call "IMAQ Create.vi"("Image Name"="Color Features", "Image Type"=w147) -> ("New Image"=w142:T1)  [unwired: 2 in, 2 out]
      n56 = call "IMAQ Create.vi"("Image Name"="Color Image 1 Modulo4", "Image Type"=w149) -> ("New Image"=w144:T1, "error out"=w143:errorcluster)  [unwired: 2 in, 1 out]
      n57 = call "IMAQ Create.vi"("Image Name"="Threshold Image", "Image Type"=w135) -> ("New Image"=w124:T1)  [unwired: 2 in, 2 out]
      n58 = call "IMAQ Create.vi"("Image Name"="Color Histograph", "Image Type"=w151) -> ("New Image"=w145:T1)  [unwired: 2 in, 2 out]
      n59 = call "IMAQ Create.vi"("Image Name"="Color Image" ("name (unnamed)"), "Image Type"=w85) -> ("New Image"=w84:T1)  [unwired: 2 in, 2 out]
      n60 = call "IMAQ Create.vi"("Image Name"="Analysis Report Image", "Image Type"=w116) -> ("New Image"=w112:T1)  [unwired: 2 in, 2 out]
      n61 = call "IMAQ Create.vi"("Image Name"="Frozen Original Image", "Image Type"=w99) -> ("New Image"=w96:T1, "error out"=w97:errorcluster)  [unwired: 2 in, 1 out]
      n62 = call "IMAQ Create.vi"("Image Name"="Backgroud", "Image Type"=w92) -> ("New Image"=w90:T1)  [unwired: 2 in, 2 out]
      n63 = call "IMAQ Create.vi"("Image Name"="Extract Image", "Image Type"=w154) -> ("New Image"=w152:T1)  [unwired: 2 in, 2 out]
      n64 = call "IMAQ Create.vi"("Image Name"="BCGLookup Image", "Image Type"=w76) -> ("New Image"=w74:T1, "error out"=w73:errorcluster)  [unwired: 2 in, 1 out]
      n65 = call "IMAQ Create.vi"("Image Name"="Threshold", "Image Type"=w131) -> ("New Image"=w120:T1)  [unwired: 2 in, 2 out]
      n66 = while {
        tunnel: w71 -> [w1062]
        tunnel: w184 -> [w1066]
        tunnel: w174 -> [w1065]
        tunnel: [w1047] -> w178
        tunnel: [w1064] -> w183
        tunnel: [w1055] -> w179
        tunnel: w100 -> [w1053]
        tunnel: w80 -> [w1050]
        tunnel: w70 -> [w1044]
        tunnel: w69 -> [w1043]
        stop <- w1059 stop-if-true
        # "Imagenes para mostrar en picture"
        # "Images para procesar en VIs"
        # "Parada si la captura\nno funciona"
        # "Pausado?"
        # "MODULO 1"
        n67 = case shown="True" w1044 {
          tunnel: w1066 -> [w1070 w1073]
          tunnel: w1065 -> [w1069 w1075]
          tunnel: [w1067 w1073] -> w1064
          tunnel: w1062 -> [w1072 w1078]
          tunnel: [w1068 w1076] -> w1055
          tunnel: [w1071 w1077] -> w1054
          tunnel: w1043 -> [_ w1074]
          frame False {
            n68 = call <vilib>:"IMAQdx Grab.vi"("error in"=w1072, "Image In"=w1069, "Session In"=w1070) -> ("error out"=w1071:errorcluster, "Image Out"=w1068:T1, "Session Out"=w1067:T21)  [unwired: 5 in, 1 out]
          }
          frame True {
            n69 = call "IMAQ Copy"("error in (no error)"=w1078, "Image Dst"=w1075, "Image Src"=w1074) -> ("error out"=w1077:errorcluster, "Image Dst Out"=w1076:T1)  [unwired: 3 in]
          }
        }
        n70 = call "IMAQ Copy"("error in (no error)"=w1054, "Image Dst"=w1053, "Image Src"=w1055) -> ("error out"=w1049:errorcluster, "Image Dst Out"=w1051:T1)  [unwired: 3 out]
        "Original Image" <- w1051
        n71 = call "IMAQ ColorImageToArray"("Image"=w1055, "error in (no error)"=w1049) -> ("Image Pixels (U32)"=w1056:u32[][], "error out"=w1048:errorcluster)  [unwired: 1 in, 2 out]
        n72 = call "Flatten Pixmap.vi"("24-bit pixmap"=w1056) -> ("image data"=w1057:T27)  [unwired: 5 in, 5 out]
        n73 = call "Draw Flattened Pixmap.vi"("image data"=w1057) -> ("new picture"=w1045:picture)  [unwired: 1 in, 7 out]
        "Source Image" <- w1045
        n74 = case shown="False" "Pause" {
          tunnel: w1051 -> [w1080 _]
          tunnel: w1045 -> [w1079 _]
          tunnel: w1050 -> [w1083 _]
          tunnel: w1049 -> [w1082 _]
          tunnel: [w1081 errorcluster {"status"=FALSE, "code"=0, "source"=""} ("error out")] -> w1046
          frame False {
            n75 = call "IMAQ Copy"("error in (no error)"=w1082, "Image Dst"=w1083, "Image Src"=w1080) -> ("error out"=w1081:errorcluster, "Image Dst Out"=→"Paused Original Image":T1)  [unwired: 3 out]
            "Paused Original Picture" <- w1079
          }
          frame True {
          }
        }
        n76 = Merge Errors(w1048, w1046) -> (w1047:errorcluster)
        n77 = Unbundle By Name(w1047) -> ("status"=w1058:bool)
        n78 = Not(x=w1058) -> (.not. x?=→"Acquiring":bool)
        n79 = property on="Source Image" class="Pict"("ZoomFactor"="Zoom") -> ()  [unwired: 2 in, 2 out]
        n80 = property on="Result Picture" class="Pict"("ZoomFactor"="Zoom") -> ()  [unwired: 2 in, 2 out]
        n81 = Or(x=w1058, y="stop") -> (x .or. y?=w1059:bool)
        "stop 2" <- w1059
        "Numeric Tab control" <- "Tab Control"
      }
      n82 = while {
        tunnel: w157 -> [w884]
        tunnel: [w845] -> w94
        tunnel: w156 -> [w843]
        tunnel: w163 -> [w880]
        tunnel: w161 -> [w877]
        tunnel: w159 -> [w873]
        tunnel: w155 -> [w844]
        tunnel: w162 -> [w841]
        tunnel: w158 -> [w839]
        tunnel: w160 -> [w835]
        tunnel: w93 -> [w823]
        tunnel: w77 -> [w785]
        stop <- w886 stop-if-true
        # "Modifica los ROIs e imagen para verse en el picture"
        # "Dibuja máscara"
        # "Si intenta dibujar un rectagulo\ncuando no hay puntos, da error;\npor eso se le pone 0 matches."
        # "Selecciona según pestaña: etiquetas Result Picture, ROIs, ratón, máscara, Match Color sin fondo, media…"
        # "Imagen final"
        # "Dibuja área contenedora de las otras"
        # "Media de la posición"
        # "Dibuja los datos en la imagen y\nenseña los cluster segun tenemos\nseleccionado en la pestaña 3"
        # "MODULO 10"
        # "Suma diferentes capas de ROIs"
        # "Dibuja los ROIs\nde los datos"
        n83 = local read "Morphology Image"() -> (w842:T1)
        n84 = call "IMAQ Copy"("error in (no error)"=w839, "Image Dst"=w873, "Image Src"=w842) -> ("error out"=w831:errorcluster, "Image Dst Out"=w874:T1)  [unwired: 3 out]
        n85 = local read "Cluster Maches Color Out"() -> (w837:T2)
        n86 = local read "Color Image"() -> (w786:T1)
        n87 = local read "Cluster Shape Report Out"() -> (w838:T3)
        n88 = local read "Cluster Particle Reports (Pixels) Out"() -> (w840:T4)
        n89 = call "IMAQ Copy"("error in (no error)"=w844, "Image Dst"=w843, "Image Src"=w786) -> ("error out"=w824:errorcluster, "Image Dst Out"=w871:T1)  [unwired: 3 out]
        n90 = Unbundle(w837) -> ("Matches Out"=w889:T28, "N. Matches Color"=w868:i32)
        n91 = Unbundle(w840) -> ("Particle Reports (Pixels)"=w883:T29, "N. Particles Report"=w865:i32)
        n92 = call "IMAQ Copy"("error in (no error)"=w841, "Image Dst"=w880, "Image Src"=w842) -> ("error out"=w832:errorcluster, "Image Dst Out"=w879:T1)  [unwired: 3 out]
        n93 = Unbundle(w838) -> ("Shape Report"=w876:T30, "N. Matches Shape"=w863:i32)
        n94 = case shown="0, Default" "Show Results" {
          tunnel: [w937 w944 w951 w959] -> w856
          tunnel: [FALSE w945 FALSE FALSE] -> w855
          tunnel: [FALSE TRUE FALSE FALSE] -> w854
          tunnel: [FALSE FALSE w952 FALSE] -> w853
          tunnel: [FALSE FALSE TRUE FALSE] -> w852
          tunnel: [FALSE FALSE FALSE w958] -> w851
          tunnel: [FALSE FALSE FALSE TRUE] -> w850
          tunnel: [w937 w944 w952 w959] -> w782
          tunnel: [w937 w945 w951 w959] -> w781
          tunnel: [w937 w944 w951 w958] -> w780
          frame 0, Default {
            w937 = TRUE
          }
          frame 1 {
            w945 = TRUE
            w944 = FALSE
          }
          frame 2 {
            w952 = TRUE
            w951 = FALSE
          }
          frame 3 {
            w958 = TRUE
            w959 = FALSE
          }
        }
        n95 = call "IMAQ Copy"("error in (no error)"=w835, "Image Dst"=w877, "Image Src"=w786) -> ("error out"=w833:errorcluster, "Image Dst Out"=w881:T1)  [unwired: 3 out]
        n96 = call "DE_MATCH _COLOR _TO _ORDER(SubVI).vi"("put in order"="Order by", "Matches In"=w889) -> ("Matches Out"=w862:T28)  [unwired: 3 out]
        n97 = call "DE_PARTICLE_REPORT_TO_ORDER(SubVI).vi"("put in order"="Order by", "Particle Reports (Pixels)"=w883) -> ("Particle Reports (Pixels) 2"=w866:T29)  [unwired: 3 out]
        n98 = call "DE_SHAPE_TO_ORDER(SubVI).vi"("put in order"="Order by", "Shape Report"=w876) -> ("Shape Report 2"=w864:T30)  [unwired: 1 in, 2 out]
        n99 = Merge Errors(w832, w833, w831) -> (w834:errorcluster)
        n100 = property on="Color Matching" class="Clust (strict)"("Visible"=w853) -> ()  [unwired: 2 in, 2 out]
        n101 = property on="Order by" class="Ring (strict)"("Visible"=w852) -> ()  [unwired: 2 in, 2 out]
        n102 = property on="Color Matching" class="Clust (strict)"("Visible"=w851) -> ()  [unwired: 2 in, 2 out]
        n103 = property on="Order by" class="Ring (strict)"("Visible"=w850) -> ()  [unwired: 2 in, 2 out]
        n104 = property on="Global Result" class="Clust (strict)"("Visible"=w856) -> ()  [unwired: 2 in, 2 out]
        n105 = property on="Particle Analysis" class="Clust (strict)"("Visible"=w855) -> ()  [unwired: 2 in, 2 out]
        n106 = property on="Order by" class="Ring (strict)"("Visible"=w854) -> ()  [unwired: 2 in, 2 out]
        n107 = Bundle("Matches Out"=w862, "N. Matches Color"=w868) -> (→"Color Matching":T2)  [unwired: 1 out]
        n108 = Bundle("Shape Report 2"=w864, "N. Matches Shape"=w863) -> (→"Particle Analysis":T31)  [unwired: 1 out]
        n109 = Bundle("Particle Reports (Pixels) 2"=w866, "N. Particles Report"=w865) -> (→"Color Matching":T32)  [unwired: 1 out]
        n110 = call "IMAQ FillImage"("Color Pixel Value"=u32 16711680, "error in (no error)"=w834, "Image Mask"=w879, "Image"=w881) -> ("error out"=w822:errorcluster, "Image Out"=w870:T1)  [unwired: 3 in, 3 out]
        n111 = call "DE_PARTICLE_REPORT_A_MATCHES(SubVI).vi"("Particle Reports (Pixels)"=w866) -> ("Matches"=w860:T28)
        n112 = call "DE_SHAPE_REPORT_A_MATCHES(SubVI).vi"("Shape Report"=w864) -> ("Matches"=w829:T28)
        n113 = case shown="True" w780 {
          tunnel: w870 -> [w890 w895]
          tunnel: w865 -> [_ w894]
          tunnel: w860 -> [_ w893]
          tunnel: [w890 w892] -> w821
          tunnel: "Show Draw Point" -> [_ w891]
          frame False {
          }
          frame True {
            n114 = call "DRAW_PATTERN_MATCHES_POSITION_ADV3(SubVI).vi"("color puntero"=u32 15728450, "Setup Show Draw"=w891, "Matches"=w893, "Number of Matches"=w894, "Image Color"=w895) -> ("Image Out"=w892:T1)  [unwired: 1 in, 5 out]
          }
        }
        n115 = case shown="True" w781 {
          tunnel: w874 -> [w897 w902]
          tunnel: w863 -> [_ w901]
          tunnel: w829 -> [_ w900]
          tunnel: [w897 w899] -> w820
          tunnel: "Show Draw Point" -> [_ w898]
          frame False {
          }
          frame True {
            n116 = call "DRAW_PATTERN_MATCHES_POSITION_ADV3(SubVI).vi"("color puntero"=u32 16711935, "Setup Show Draw"=w898, "Matches"=w900, "Number of Matches"=w901, "Image Color"=w902) -> ("Image Out"=w899:T1)  [unwired: 1 in, 5 out]
          }
        }
        n117 = case shown="True" w782 {
          tunnel: w871 -> [w904 w909]
          tunnel: w868 -> [_ w908]
          tunnel: w862 -> [_ w907]
          tunnel: [w904 w906] -> w849
          tunnel: "Show Draw Point" -> [_ w905]
          frame False {
          }
          frame True {
            n118 = call "DRAW_PATTERN_MATCHES_POSITION_ADV3(SubVI).vi"("color puntero"=u32 204, "Setup Show Draw"=w905, "Matches"=w907, "Number of Matches"=w908, "Image Color"=w909) -> ("Image Out"=w906:T1)  [unwired: 1 in, 5 out]
          }
        }
        n119 = local read "Rect Out"() -> (w848:T5)
        n120 = for {
          tunnel: w862 -> [w1037] mode=indexing
          tunnel: [w1036] -> w801
          tunnel: [w1035] -> w793
          n121 = Unbundle By Name(w1037) -> ("Position"=w1036:cluster{"x":sgl, "y":sgl}, "Bounding Box"=w1035:cluster{"x":sgl, "y":sgl}[])
        }
        n122 = for {
          tunnel: w860 -> [w1034] mode=indexing
          tunnel: [w1033] -> w815
          tunnel: [w1032] -> w795
          n123 = Unbundle By Name(w1034) -> ("Position"=w1033:cluster{"x":sgl, "y":sgl}, "Bounding Box"=w1032:cluster{"x":sgl, "y":sgl}[])
        }
        n124 = for {
          tunnel: w829 -> [w1039] mode=indexing
          tunnel: [w1041] -> w800
          tunnel: [w1040] -> w859
          tunnel: [w1038] -> w794
          n125 = Unbundle By Name(w1039) -> ("Position"=w1041:cluster{"x":sgl, "y":sgl}, "Scale"=w1040:sgl, "Bounding Box"=w1038:cluster{"x":sgl, "y":sgl}[])
        }
        n126 = call "IMAQ Overlay Rectangle"("Color"="Pen Color", "error in (no error)"=w824, "Rectangle"=w848, "Image"=w849) -> ("error out"=w816:errorcluster, "Image Out"=w817:T1)  [unwired: 2 in, 4 out]
        n127 = call "IMAQ Copy"("error in (no error)"=w823, "Image Dst"=w884, "Image Src"=w817) -> ("error out"=w878:errorcluster, "Image Dst Out"=w885:T1)  [unwired: 3 out]
        n128 = call "IMAQ Copy Overlay"("error in (no error)"=w878, "Image Dst"=w885, "Image Src"=w821) -> ("error out"=w830:errorcluster, "Image Dst Out"=w872:T1)  [unwired: 1 in, 6 out]
        n129 = Equal To 0?(x=w815) -> (x = 0?=w814:cluster{"x":bool, "y":bool})
        n130 = Equal To 0?(x=w801) -> (x = 0?=w803:cluster{"x":bool, "y":bool})
        n131 = call "XYMEAN(SubVI).vi"("Object Size"=w859, "Position Analysis Report"=w815, "Position Match Shape"=w800, "Position Match Color"=w801) -> ("Result"=w783:T33)
        "Global Result" <- w783
        n132 = Equal To 0?(x=w800) -> (x = 0?=w805:cluster{"x":bool, "y":bool})
        n133 = local read "Numeric Tab control"() -> (w858:i32)
        n134 = Cluster To Array(cluster=w803) -> (array=w802:bool[])
        n135 = Cluster To Array(cluster=w814) -> (array=w813:bool[])
        n136 = Cluster To Array(cluster=w805) -> (array=w804:bool[])
        n137 = And Array Elements(Boolean array=w802) -> (logical AND=w799:bool)
        n138 = call "IMAQ Copy Overlay"("error in (no error)"=w830, "Image Dst"=w872, "Image Src"=w820) -> ("error out"=w847:errorcluster, "Image Dst Out"=w846:T1)  [unwired: 1 in, 6 out]
        n139 = And Array Elements(Boolean array=w804) -> (logical AND=w798:bool)
        n140 = And Array Elements(Boolean array=w813) -> (logical AND=w797:bool)
        n141 = call "IMAQ Copy Overlay"("error in (no error)"=w822, "Image Dst"=w821, "Image Src"=w820) -> ("error out"=w819:errorcluster, "Image Dst Out"=w818:T1)  [unwired: 1 in, 6 out]
        n142 = Boolean To (0,1)(Boolean=w797) -> (0, 1=w809:i16)
        n143 = Boolean To (0,1)(Boolean=w799) -> (0, 1=w812:i16)
        n144 = Boolean To (0,1)(Boolean=w798) -> (0, 1=w810:i16)
        n145 = Number To Decimal String(number=w809) -> (decimal integer string=w807:string)  [unwired: 1 out]
        n146 = Number To Decimal String(number=w812) -> (decimal integer string=w811:string)  [unwired: 1 out]
        n147 = Number To Decimal String(number=w810) -> (decimal integer string=w808:string)  [unwired: 1 out]
        n148 = Concatenate Strings(w811, w808, w807) -> (w806:string)
        n149 = case shown="\"100\"" w806 {
          tunnel: [w912 w918 w922 w926 w928 w932 w934 cluster{"x":sgl, "y":sgl}[] [] ("Bounding Box Out")] -> w796
          tunnel: w795 -> [w915 _ w923 _ w929 _ w934 _]
          tunnel: w794 -> [w916 w920 _ _ w930 w932 _ _]
          tunnel: w793 -> [w914 w919 w924 w926 _ _ _ _]
          tunnel: [1 1 1 1 1 1 1 0] -> w792
          frame "000" {
            n150 = call "BOX_TO_BOX(SubVI).vi"("Bounding Box 2"=w915, "Bounding Box 1"=w916) -> ("Bounding Box Out"=w913:cluster{"x":sgl, "y":sgl}[])
            n151 = call "BOX_TO_BOX(SubVI).vi"("Bounding Box 2"=w913, "Bounding Box 1"=w914) -> ("Bounding Box Out"=w912:cluster{"x":sgl, "y":sgl}[])
          }
          frame "001" {
            n152 = call "BOX_TO_BOX(SubVI).vi"("Bounding Box 2"=w920, "Bounding Box 1"=w919) -> ("Bounding Box Out"=w918:cluster{"x":sgl, "y":sgl}[])
          }
          frame "010" {
            n153 = call "BOX_TO_BOX(SubVI).vi"("Bounding Box 2"=w923, "Bounding Box 1"=w924) -> ("Bounding Box Out"=w922:cluster{"x":sgl, "y":sgl}[])
          }
          frame "011" {
          }
          frame "100" {
            n154 = call "BOX_TO_BOX(SubVI).vi"("Bounding Box 2"=w929, "Bounding Box 1"=w930) -> ("Bounding Box Out"=w928:cluster{"x":sgl, "y":sgl}[])
          }
          frame "101" {
          }
          frame "110" {
          }
          frame "111", Default {
          }
        }
        n155 = case shown="2" w858 {
          tunnel: w819 -> [w968 w976 w993 w1013]
          tunnel: w818 -> [_ w975 _ _]
          tunnel: w817 -> [_ _ w984 _]
          tunnel: w816 -> [w966 w977 w982 w1014]
          tunnel: [w968 w976 w993 w1013] -> w827
          tunnel: [w965 w975 w985 w1011] -> w836
          tunnel: w847 -> [w967 w978 w992 w1012]
          tunnel: w846 -> [_ _ _ w1018]
          tunnel: w783 -> [_ _ _ w1015]
          tunnel: [w967 w978 w992 w1012] -> w826
          tunnel: [w966 w977 w981 w1014] -> w825
          tunnel: w796 -> [_ _ _ w1010]
          tunnel: w792 -> [_ _ _ w1008]
          tunnel: w785 -> [_ _ w983 _]
          tunnel: "Show Draw Point" -> [_ _ _ w1009]
          frame 0, Default {
            n156 = local read "Color Image"() -> (w965:T1)
            n157 = property on="Result Picture" class="Pict"("Caption.Text"="Color Processing") -> ()  [unwired: 2 in, 2 out]
          }
          frame 1 {
            n158 = property on="Result Picture" class="Pict"() -> ("Mouse"=w970:T34)  [unwired: 2 in, 2 out]
            n159 = Unbundle By Name(w970) -> ("Mouse Position"=w972:cluster{"X":i32, "Y":i32})
            n160 = property on="Result Picture" class="Pict"("Caption.Text"="Particle Analysis" ("Label.Text")) -> ()  [unwired: 2 in, 2 out]
            n161 = Greater Than 0?(x=w972) -> (x > 0?=w971:cluster{"X":bool, "Y":bool})
            n162 = Cluster To Array(cluster=w971) -> (array=w973:bool[])
            n163 = And Array Elements(Boolean array=w973) -> (logical AND=w974:bool)
            n164 = case shown="True" w974 {
              frame False {
                n165 = call "Set_Cursor_(IconPict).vi"() -> ()  [unwired: 3 in, 9 out]
              }
              frame True {
                n166 = call "Set_Cursor_(IconPict).vi"("icon"=u16 26) -> ()  [unwired: 2 in, 9 out]
              }
            }
          }
          frame 2 {
            n167 = property on="Result Picture" class="Pict"() -> ("Mouse"=w991:T34)  [unwired: 2 in, 2 out]
            n168 = local read "Background Subtraction"() -> (w986:bool)
            n169 = case shown="False" w986 {
              tunnel: [w1000 w1004] -> w985
              tunnel: w984 -> [w996 w1004]
              tunnel: w983 -> [w1001 _]
              tunnel: w982 -> [w995 w1003]
              tunnel: [w997 w1003] -> w981
              frame False {
                n170 = local read "BCG Image"() -> (w1002:T1)
                n171 = call "IMAQ Copy"("error in (no error)"=w995, "Image Dst"=w1001, "Image Src"=w1002) -> ("error out"=w998:errorcluster, "Image Dst Out"=w999:T1)  [unwired: 3 out]
                n172 = call "IMAQ Copy Overlay"("error in (no error)"=w998, "Image Dst"=w999, "Image Src"=w996) -> ("error out"=w997:errorcluster, "Image Dst Out"=w1000:T1)  [unwired: 1 in, 6 out]
              }
              frame True {
              }
            }
            n173 = Unbundle By Name(w991) -> ("Mouse Position"=w989:cluster{"X":i32, "Y":i32})
            n174 = Greater Than 0?(x=w989) -> (x > 0?=w990:cluster{"X":bool, "Y":bool})
            n175 = Cluster To Array(cluster=w990) -> (array=w988:bool[])
            n176 = And Array Elements(Boolean array=w988) -> (logical AND=w987:bool)
            n177 = property on="Result Picture" class="Pict"("Caption.Text"="Object Matching" ("Label.Text")) -> ()  [unwired: 2 in, 2 out]
            n178 = case shown="False" w987 {
              frame False {
                n179 = call "Set_Cursor_(IconPict).vi"() -> ()  [unwired: 3 in, 9 out]
              }
              frame True {
                n180 = call "Set_Cursor_(IconPict).vi"("icon"=u16 27) -> ()  [unwired: 2 in, 9 out]
              }
            }
          }
          frame 3 {
            n181 = for {
              N: 1 -> [_]
              tunnel: [w1031] -> w1016 mode=indexing
              tunnel: w1015 -> [w1029]
              tunnel: w1010 -> [w1028]
              n182 = Unbundle(w1029) -> ("Position"=w1027:cluster{"X":sgl, "Y":sgl})  [unwired: 3 out]
              n183 = Bundle By Name(cluster=T23 {"Position"={"x"=0.0, "y"=0.0}, "Angle"=0.0, "Scale"=0.0, "Score"=0.0, "Bounding Box"=[]}, "Position"=w1027, "Bounding Box"=w1028) -> (w1031:T23)
            }
            n184 = local read "Show Results"() -> (w1006:u16)
            n185 = property on="Result Picture" class="Pict"("Caption.Text"="Report") -> ()  [unwired: 2 in, 2 out]
            n186 = Equal To 0?(x=w1006) -> (x = 0?=w1007:bool)
            n187 = case shown="False" w1007 {
              tunnel: w1018 -> [w1020 w1025]
              tunnel: w1016 -> [_ w1024]
              tunnel: [w1020 w1023] -> w1011
              tunnel: w1009 -> [_ w1022]
              tunnel: w1008 -> [_ w1021]
              frame False {
              }
              frame True {
                n188 = call "DRAW_PATTERN_MATCHES_POSITION_ADV3(SubVI).vi"("color puntero"=u32 16751616, "Setup Show Draw"=w1022, "Matches"=w1024, "Number of Matches"=w1021, "Image Color"=w1025) -> ("Image Out"=w1023:T1)  [unwired: 1 in, 5 out]
              }
            }
          }
        }
        n189 = Merge Errors(w827, w826, w825) -> (w828:errorcluster)
        n190 = call "IMAQ Merge Overlay"("error in (no error)"=w828, "Image Src"=w836) -> ("error out"=w787:errorcluster, "Image Dst Out"=w788:T1)  [unwired: 3 in, 5 out]
        n191 = call "IMAQ ColorImageToArray"("Image"=w788, "error in (no error)"=w787) -> ("Image Pixels (U32)"=w791:u32[][], "error out"=w845:errorcluster)  [unwired: 1 in, 2 out]
        n192 = call "Flatten Pixmap.vi"("24-bit pixmap"=w791) -> ("image data"=w790:T27)  [unwired: 5 in, 5 out]
        n193 = local read "stop 2"() -> (w886:bool)
        n194 = call "Draw Flattened Pixmap.vi"("image data"=w790) -> ("new picture"=→"Result Picture":picture)  [unwired: 1 in, 7 out]
      }
      n195 = while {
        tunnel: [w236] -> w182
        tunnel: [w231] -> w95
        tunnel: [w235] -> w181
        tunnel: [w234] -> w180
        tunnel: [w233] -> w177
        tunnel: w97 -> [w225]
        tunnel: w152 -> [w224]
        tunnel: w142 -> [w223]
        tunnel: w143 -> [w222]
        tunnel: w144 -> [w221]
        tunnel: w145 -> [w220]
        tunnel: w123 -> [w219]
        tunnel: w122 -> [w218]
        tunnel: w121 -> [w217]
        tunnel: w120 -> [w216]
        tunnel: w124 -> [w215]
        tunnel: w125 -> [w204]
        tunnel: w126 -> [w214]
        tunnel: w127 -> [w213]
        tunnel: w112 -> [w212]
        tunnel: w115 -> [w211]
        tunnel: w113 -> [w210]
        tunnel: w114 -> [w209]
        tunnel: w105 -> [w208]
        tunnel: w104 -> [w207]
        tunnel: w107 -> [w206]
        tunnel: w106 -> [w205]
        tunnel: w96 -> [w203]
        tunnel: w90 -> [w201]
        tunnel: w87 -> [w200]
        tunnel: w84 -> [w199]
        tunnel: [w198] -> w83
        tunnel: w74 -> [w197]
        tunnel: w73 -> [w196]
        stop <- w232 stop-if-true
        # "Activar Modulo?"
        # "Activar Modulo?"
        # "Activar Modulo?"
        # "Activar Modulo?"
        # "Activar Modulo?"
        # "Activar Modulo?"
        n196 = case shown="True" TRUE {
          tunnel: [errorcluster {"status"=FALSE, "code"=0, "source"=""} ("error out") w726] -> w231
          tunnel: w208 -> [_ w725]
          tunnel: w207 -> [_ w724]
          tunnel: w206 -> [_ w723]
          tunnel: w205 -> [_ w722]
          frame False {
          }
          frame True {
            n197 = for {
              N: 1 -> [_]
              tunnel: w724 -> [w744]
              tunnel: w722 -> [w740]
              tunnel: w725 -> [w746]
              tunnel: [w735] -> w726
              tunnel: w723 -> [w747]
              w733 = T35 4 items=["Any", "Calibration", "Overlay", "Grayscale Template", "Color Template", "Geometric Template", "Custom Data", "Golden Template"] ("Vision Info")
              # "Quieres busqueda en imagen original o con?"
              # "MODULO 7"
              # "Hay Template?"
              # "Busqueda Template"
              n198 = local read "Extract Image"() -> (w739:T1)
              n199 = local read "Background Subtraction"() -> (w728:bool)
              n200 = case shown="True" "Learn Template" {
                tunnel: w744 -> [w760 w765]
                tunnel: w746 -> [_ w770]
                tunnel: [w761 w763] -> w734
                tunnel: [w760 w762] -> w745
                tunnel: w739 -> [_ w764]
                frame False {
                  # "Template en memoria"
                  n201 = local read "Image Template Out"() -> (w761:T1)
                }
                frame True {
                  # "Aprende Template"
                  n202 = call "IMAQ Copy"("error in (no error)"=w765, "Image Dst"=w770, "Image Src"=w764) -> ("error out"=w768:errorcluster, "Image Dst Out"=w769:T1)  [unwired: 3 out]
                  n203 = Unbundle("Learn Control") -> ("Saturation Threshold"=w776:i32, "Ignore Black and White"=w777:u32, "Feature Mode"=w778:u32, "Ignore Color Spectra"=w774:dbl[][], "Learn Mode"=w775:u16)
                  n204 = call "IMAQ Setup Learn Color Pattern"("Saturation Threshold"=w776, "Ignore Color Spectra"=w774, "error in (no error)"=w768, "Ignore Black and White"=w777, "Feature Mode"=w778, "Learn Mode"=w775) -> ("error out"=w771:errorcluster, "Learn Color Pattern Setup Data"=w773:string)  [unwired: 4 out]
                  n205 = call "IMAQ Learn Color Pattern"("error in (no error)"=w771, "Learn Color Pattern Setup Data"=w773, "Image"=w769) -> ("error out"=w767:errorcluster, "Template Image Out"=w763:T1)  [unwired: 7 out]
                  "Image Template Out" <- w763
                  n206 = property on="Learn Template" class="Bool (strict)"(error in=w767, "Value"=FALSE ("Template")) -> (error out=w762:errorcluster)  [unwired: 1 in, 1 out]
                }
              }
              n207 = case shown="False" w728 {
                tunnel: [w748 w749] -> w727
                frame False {
                  n208 = local read "BCG Image"() -> (w748:T1)
                }
                frame True {
                  n209 = local read "Color Image"() -> (w749:T1)
                }
              }
              n210 = call "IMAQ Copy"("error in (no error)"=w740, "Image Dst"=w747, "Image Src"=w727) -> ("error out"=w736:errorcluster, "Image Dst Out"=w737:T1)  [unwired: 3 out]
              n211 = Merge Errors(w736, w745) -> (w731:errorcluster)
              n212 = call "IMAQ Is Vision Info Present 2"("error in (no error)"=w731, "Vision Info"=w733, "Image"=w734) -> ("error out"=w730:errorcluster, "Present?"=w729:bool, "Image (duplicate)"=w732:T1)  [unwired: 6 out]
              n213 = case shown="False" w729 {
                tunnel: w732 -> [_ w758]
                tunnel: w730 -> [w751 w757]
                tunnel: w737 -> [_ w756]
                tunnel: [w750 w755] -> w735
                tunnel: [_ w754] -> w743
                tunnel: [0 ("Number of Matches Out") w753] -> w742
                frame False {
                  # "Elimina error cuando\nno se ha hecho ninguna\nprimera búsqueda"
                  n214 = call "Clear Errors.vi"("error in (no error)"=w751) -> ("error out"=w750:errorcluster)  [unwired: 6 out]
                }
                frame True {
                  n215 = call "SEARCH(SubVI).vi"("Image In"=w756, "search control In"="Search Control", "Image Temaplate In"=w758, "error in"=w757) -> ("Matches Out"=w754:T28, "Number of Matches Out"=w753:i32, "error out"=w755:errorcluster)  [unwired: 2 in, 7 out]
                }
              }
              n216 = Bundle("Matches Out"=w743, "Number of Matches Out"=w742) -> (→"Cluster Maches Color Out":T36)  [unwired: 1 out]
            }
          }
        }
        n217 = case shown="True" TRUE {
          tunnel: w201 -> [_ w243]
          tunnel: w200 -> [_ w242]
          tunnel: w199 -> [_ w241]
          tunnel: [errorcluster {"status"=FALSE, "code"=0, "source"=""} ("error out") w240] -> w198
          tunnel: w197 -> [_ w239]
          tunnel: w196 -> [_ w238]
          frame False {
          }
          frame True {
            n218 = for {
              N: 1 -> [_]
              tunnel: w243 -> [w258]
              tunnel: w242 -> [w257]
              tunnel: w241 -> [w256]
              tunnel: [w253] -> w240
              tunnel: w239 -> [w250]
              tunnel: w238 -> [w246]
              # "Pausado?"
              # "MODULO 3"
              n219 = local read "Pause"() -> (w251:bool)
              n220 = case shown="False" w251 {
                tunnel: [w261 w262] -> w248
                frame False {
                  n221 = local read "Original Image"() -> (w261:T1)
                }
                frame True {
                  n222 = local read "Paused Original Image"() -> (w262:T1)
                }
              }
              n223 = call "IMAQ ColorBCGLookup"("Blue BCG Values"="Background Correction", "Green BCG Values"="Background Correction", "error in (no error)"=w246, "Red BCG Values"="Background Correction", "Image Dst"=w250, "Image Src"=w248) -> ("error out"=w247:errorcluster, "Image Dst Out"=w249:T1)  [unwired: 1 in, 3 out]
              "BCG Image" <- w249
              n224 = call "Boolean Trigger__ogtk.vi"("Boolean Input"="Subtraction") -> ("Rising Edge"=w259:bool)  [unwired: 2 out]
              n225 = case shown="True" "Subtraction" {
                tunnel: w257 -> [_ w277]
                tunnel: w259 -> [_ w273]
                tunnel: w249 -> [w263 w270]
                tunnel: w247 -> [w264 w269]
                tunnel: [w264 w268] -> w255
                tunnel: [w263 w267] -> w254
                tunnel: w258 -> [_ w266]
                frame False {
                }
                frame True {
                  w274 = T26 4 items=["Grayscale (U8)", "Grayscale (I16)", "Grayscale (SGL)", "Complex (CSG)", "RGB (U32)", "HSL (U32)", "RGB (U64)"] ("Image Type")
                  # "Filtro de eliminacion de fondo; captura el fondo de ese momento y lo resta al actual"
                  n226 = case shown="True" w273 {
                    tunnel: w270 -> [_ w286]
                    tunnel: [w281 w284] -> w272
                    tunnel: w266 -> [_ w285]
                    tunnel: [w280 w283] -> w271
                    tunnel: w269 -> [w280 w282]
                    frame False {
                      n227 = local read "Backgroud In"() -> (w281:T1)
                    }
                    frame True {
                      # "almacena el fondo en memoria"
                      n228 = call "IMAQ Copy"("error in (no error)"=w282, "Image Dst"=w285, "Image Src"=w286) -> ("error out"=w283:errorcluster, "Image Dst Out"=w284:T1)  [unwired: 3 out]
                      "Backgroud In" <- w284
                    }
                  }
                  n229 = call "IMAQ Copy"("error in (no error)"=w269, "Image Dst"=w277, "Image Src"=w270) -> ("error out"=w265:errorcluster, "Image Dst Out"=w275:T1)  [unwired: 3 out]
                  n230 = call "IMAQ Copy"("error in (no error)"=w271, "Image Dst"=w266, "Image Src"=w272) -> ("error out"=w276:errorcluster, "Image Dst Out"=w279:T1)  [unwired: 3 out]
                  n231 = Merge Errors(w265, w276) -> (w278:errorcluster)
                  n232 = call "ELIMINA_FONDO_SIN BUFFER(subVI).vi"("Image Type"=w274, "error in"=w278, "Backgroud In"=w279, "Image In"=w275) -> ("error out"=w268:errorcluster, "Image 1 Add 2"=w267:T1)  [unwired: 6 out]
                }
              }
              n233 = call "IMAQ Copy"("error in (no error)"=w255, "Image Dst"=w256, "Image Src"=w254) -> ("error out"=w253:errorcluster, "Image Dst Out"=→"Color Image":T1)  [unwired: 3 out]
            }
          }
        }
        n234 = case shown="True" TRUE {
          tunnel: [errorcluster {"status"=FALSE, "code"=0, "source"=""} ("error out") w292] -> w233
          tunnel: w225 -> [_ w290]
          tunnel: w224 -> [_ w289]
          tunnel: w203 -> [_ w288]
          frame False {
          }
          frame True {
            n235 = for {
              N: 1 -> [_]
              tunnel: [w312] -> w292
              tunnel: w289 -> [w311]
              tunnel: w290 -> [w309]
              tunnel: w288 -> [w308]
              shift-right: [w295] -> _
              shift-left: _ -> [w294]
              # "Precisión del\nNew Square"
              # "Imagen a la que se le hace el ROI"
              # "Extrae el rectángulo y lo muestra"
              # "Transfoma dos puntos dados por el ratón\nen coordenadas para dibujar un rectángulo"
              # "MODULO 2"
              n236 = local read "Numeric Tab control"() -> (w307:i32)
              n237 = case shown="2" w307 {
                tunnel: [_ _ w332 _] -> w305
                frame 0, Default {
                }
                frame 1 {
                }
                frame 2 {
                  n238 = property on="Result Picture" class="Pict"() -> ("Mouse"=w332:T34)  [unwired: 2 in, 2 out]
                }
                frame 3 {
                }
              }
              n239 = case shown="False" "Background Subtraction" {
                tunnel: [w330 w331] -> w300
                frame False {
                  n240 = local read "BCG Image"() -> (w330:T1)
                }
                frame True {
                  n241 = local read "Color Image"() -> (w331:T1)
                }
              }
              n242 = Unbundle By Name(w305) -> ("Mouse Position"=w297:cluster{"X":i32, "Y":i32}, "Mouse Modifiers.Button Down"=w296:bool)
              n243 = case shown="True" w296 {
                tunnel: w297 -> [w314 w316]
                tunnel: w294 -> [_ w317]
                tunnel: [w314 w317] -> w295
                tunnel: [T22 {"[0]"=0, "[0]"=0, "[1]"=0, "[1]"=0} w315] -> w293
                frame False {
                }
                frame True {
                  n244 = Unbundle By Name(w317) -> ("X"=w325:i32, "Y"=w322:i32)
                  n245 = Unbundle By Name(w316) -> ("X"=w318:i32, "Y"=w321:i32)
                  n246 = Max & Min(x=w325, y=w318) -> (max(x,y)=w323:i32, min(x,y)=w324:i32)
                  n247 = Max & Min(x=w322, y=w321) -> (max(x,y)=w319:i32, min(x,y)=w320:i32)
                  n248 = Bundle(w324, w320, w323, w319) -> (w315:cluster{i32, i32, i32, i32})  [unwired: 1 out]
                }
              }
              "Rect Out" <- w293
              n249 = Not Equal To 0?(x=w293) -> (x != 0?=w302:T37)
              n250 = Cluster To Array(cluster=w302) -> (array=w301:bool[])
              n251 = And Array Elements(Boolean array=w301) -> (logical AND=w299:bool)
              n252 = call "IMAQ Copy"("error in (no error)"=w309, "Image Dst"=w308, "Image Src"=w300) -> ("error out"=w310:errorcluster, "Image Dst Out"=w306:T1)  [unwired: 3 out]
              n253 = case shown="True" w299 {
                selector: w299 -> [_ w329]
                tunnel: ["ROI Box" w328] -> w303
                tunnel: w293 -> [_ w328]
                tunnel: [w327 w329] -> w298
                frame False {
                  n254 = call-poly "Data Changed__ogtk.vi"("Variant"="ROI Box") -> ("Changed"=w327:bool)
                }
                frame True {
                  n255 = local write "ROI Box"(w328) -> ()
                }
              }
              n256 = case shown="True" w298 {
                tunnel: [w333 w336] -> w312
                tunnel: w311 -> [_ w342]
                tunnel: w310 -> [w333 w343]
                tunnel: w306 -> [_ w341]
                tunnel: w303 -> [_ w340]
                frame False {
                  n257 = local read "Extract Picture"() -> (w334:picture)
                  n258 = local write "Extract Picture"(w334) -> ()
                }
                frame True {
                  n259 = Cluster To Array(cluster=w340) -> (array=w344:dbl[])
                  n260 = call "IMAQ Extract"("Optional Rectangle"=w344, "error in (no error)"=w343, "Image Dst"=w342, "Image Src"=w341) -> ("error out"=w337:errorcluster, "Image Dst Out"=w335:T1)  [unwired: 2 in, 4 out]
                  "Extract Image" <- w335
                  n261 = call "IMAQ ColorImageToArray"("Image"=w335, "error in (no error)"=w337) -> ("Image Pixels (U32)"=w338:u32[][], "error out"=w336:errorcluster)  [unwired: 1 in, 2 out]
                  n262 = call "Flatten Pixmap.vi"("24-bit pixmap"=w338) -> ("image data"=w339:T27)  [unwired: 5 in, 5 out]
                  n263 = call "Draw Flattened Pixmap.vi"("image data"=w339) -> ("new picture"=→"Extract Picture":picture)  [unwired: 1 in, 7 out]
                }
              }
            }
          }
        }
        n264 = case shown="True" TRUE {
          tunnel: [errorcluster {"status"=FALSE, "code"=0, "source"=""} ("error IO") w562] -> w236
          tunnel: w223 -> [_ w560]
          tunnel: w222 -> [_ w559]
          tunnel: w221 -> [_ w558]
          tunnel: w220 -> [_ w557]
          frame False {
          }
          frame True {
            n265 = for {
              N: 1 -> [_]
              tunnel: [w571] -> w562
              tunnel: w558 -> [w570]
              tunnel: w560 -> [w567]
              tunnel: w557 -> [w566]
              tunnel: w559 -> [w564]
              # "MODULO 4"
              n266 = local read "Color Image"() -> (w563:T1)
              n267 = local read "Numeric Tab control"() -> (w565:i32)
              n268 = call "IMAQ Copy"("error in (no error)"=w564, "Image Dst"=w570, "Image Src"=w563) -> ("error out"=w568:errorcluster, "Image Dst Out"=w569:T1)  [unwired: 3 out]
              n269 = case shown="No Error" w568 {
                selector: w568 -> [w596 w656]
                tunnel: [w598 w656] -> w571
                tunnel: w569 -> [w595 _]
                tunnel: w567 -> [w599 _]
                tunnel: w566 -> [w597 _]
                tunnel: w565 -> [w585 _]
                frame No Error {
                  # "El refresco de Color learn es solo cuando se esta en la pestaña correspondiente y ademas se aprieta algun controlador."
                  # "El refresco del histograma se produce al cambiar de\nColor Mode o manualmente, para no consumir recursos."
                  n270 = Equal To 0?(x=w585) -> (x = 0?=w574:bool)
                  n271 = call "IMAQ Copy"("error in (no error)"=w596, "Image Dst"=w599, "Image Src"=w595) -> ("error out"=w594:errorcluster, "Image Dst Out"=w593:T1)  [unwired: 3 out]
                  n272 = call "IMAQ Copy"("error in (no error)"=w596, "Image Dst"=w597, "Image Src"=w595) -> ("error out"=w584:errorcluster, "Image Dst Out"=w592:T1)  [unwired: 3 out]
                  n273 = call-poly "Data Changed__ogtk.vi"("I32"="Saturation Threshold") -> ("Changed"=w575:bool)
                  n274 = local read "Refresh"() -> (w576:bool)
                  n275 = call-poly "Data Changed__ogtk.vi"("U32"="Color Sensitivity") -> ("Changed"=w573:bool)
                  n276 = Compound Arithmetic op=OR(w573, w575, w576) -> (w572:bool)
                  n277 = And(x=w574, y=w572) -> (x .and. y?=w577:bool)
                  n278 = case shown="True" w577 {
                    tunnel: w594 -> [w610 w615]
                    tunnel: w593 -> [_ w614]
                    tunnel: [w610 w613] -> w591
                    tunnel: "Saturation Threshold" -> [_ w612]
                    tunnel: "Color Sensitivity" -> [_ w611]
                    frame False {
                    }
                    frame True {
                      # "Format the color spectrum to display it in the appropriate graph."
                      n279 = call "IMAQ ColorLearn"("Image"=w614, "Color Sensitivity"=w611, "Learn Saturation Threshold"=w612, "error in (no error)"=w615) -> ("Color Spectrum"=w619:dbl[], "error out"=w613:errorcluster)  [unwired: 1 in, 3 out]
                      n280 = case shown="0, Default" w611 {
                        tunnel: w619 -> [w624 w636 w648]
                        tunnel: [TRUE FALSE FALSE] -> w618
                        tunnel: [FALSE TRUE FALSE] -> w617
                        tunnel: [FALSE FALSE TRUE] -> w616
                        frame 0, Default {
                          n281 = Initialize Array(0.0 ("Element Data"), 16) -> (w625:dbl[])
                          n282 = for {
                            tunnel: w624 -> [w631] mode=indexing
                            tunnel: [w629] -> w620 mode=indexing
                            tunnel: w625 -> [w628]
                            i -> [w630]
                            n283 = Replace Array Subset(array=w628, new element=w631, index=w630) -> (w629:dbl[])
                          }
                          "Color Spectrum - Low Sensitivity" <- w620
                        }
                        frame 1 {
                          n284 = Initialize Array(0.0 ("Element Data"), 30) -> (w637:dbl[])
                          n285 = for {
                            tunnel: w636 -> [w643] mode=indexing
                            tunnel: [w641] -> w632 mode=indexing
                            tunnel: w637 -> [w640]
                            i -> [w642]
                            n286 = Replace Array Subset(array=w640, new element=w643, index=w642) -> (w641:dbl[])
                          }
                          "Medium Sensitivity" <- w632
                        }
                        frame 2 {
                          n287 = Initialize Array(0.0 ("Element Data"), 58) -> (w649:dbl[])
                          n288 = for {
                            tunnel: w648 -> [w655] mode=indexing
                            tunnel: [w653] -> w644 mode=indexing
                            tunnel: w649 -> [w652]
                            i -> [w654]
                            n289 = Replace Array Subset(array=w652, new element=w655, index=w654) -> (w653:dbl[])
                          }
                          "High Sensitivity" <- w644
                        }
                      }
                      n290 = property on="Color Spectrum - Low Sensitivity" class="WFGraph (strict)"("Visible"=w618) -> ()  [unwired: 2 in, 2 out]
                      n291 = property on="Medium Sensitivity" class="WFGraph (strict)"("Visible"=w617) -> ()  [unwired: 2 in, 2 out]
                      n292 = property on="High Sensitivity" class="WFGraph (strict)"("Visible"=w616) -> ()  [unwired: 2 in, 2 out]
                    }
                  }
                  n293 = property on="Threshold Color Mode" class="Ring (strict)"() -> ("Value"=w588:u16)  [unwired: 2 in, 2 out]
                  n294 = control-ref of="Color Mode"() -> (w586:refnum<vi>)
                  n295 = control-ref of="Threshold Color Mode"() -> (w587:refnum<vi>)
                  n296 = call "TWO_BOTTON_TO_ONE(SubVI).vi"(1:"Boton 2"=w587, 2:"Boton 2"=w588, 3:"Boton 1"="Color Mode", 4:"Boton 1"=w586) -> ("Value"=w581:u16)
                  n297 = call-poly "Data Changed__ogtk.vi"("U16"=w581) -> ("Changed"=w583:bool)
                  n298 = Or(x=w583, y="Refresh") -> (x .or. y?=w580:bool)
                  n299 = case shown="False" w580 {
                    tunnel: w592 -> [_ w609]
                    tunnel: [w601 w604] -> w590
                    tunnel: w584 -> [w601 w603]
                    tunnel: w581 -> [_ w602]
                    frame False {
                      n300 = local read "Histogram"() -> (w600:T7)
                      n301 = local write "Histogram"(w600) -> ()
                    }
                    frame True {
                      n302 = call "IMAQ ColorHistograph"("Color Mode"=w602, "Image Src"=w609, "error in (no error)"=w603) -> ("Red or Hue Histogram Graph"=w607:T38, "Green or Sat Histogram Graph"=w606:T38, "Blue or Luma or Val or Inten Histogram Graph"=w605:T38, "error out"=w604:errorcluster)  [unwired: 2 in, 1 out]
                      n303 = Build Array(w607, w606, w605) -> (→"Histogram":T7)
                    }
                  }
                  n304 = Merge Errors(w590, w591) -> (w598:errorcluster)
                }
                frame Error {
                }
              }
            }
          }
        }
        n305 = case shown="True" TRUE {
          tunnel: [errorcluster {"status"=FALSE, "code"=0, "source"=""} ("error IO") w357] -> w234
          tunnel: w219 -> [_ w355]
          tunnel: w218 -> [_ w354]
          tunnel: w217 -> [_ w353]
          tunnel: w216 -> [_ w352]
          tunnel: w215 -> [_ w351]
          tunnel: w204 -> [_ w350]
          tunnel: w214 -> [_ w349]
          tunnel: w213 -> [_ w348]
          tunnel: w212 -> [_ w347]
          frame False {
          }
          frame True {
            n306 = for {
              N: 1 -> [_]
              tunnel: w353 -> [w382]
              tunnel: w352 -> [w385]
              tunnel: w355 -> [w383]
              tunnel: w351 -> [w378]
              tunnel: w354 -> [w365]
              tunnel: w350 -> [w371]
              tunnel: w348 -> [w372]
              tunnel: w349 -> [w370]
              tunnel: w347 -> [w369]
              tunnel: [w361] -> w357
              # "Mostras controladores\nde alguno VIs"
              # "PROCESAMIENTO DE LAS PARTICULAS BINARIO (MORPHOLOGY)------->"
              # "PROCESAMIENTO DE LA CAPTURA  THRESHOLD   ------7"
              # "ANALISIS PARTICULAS BINARIO  --------------->"
              # "MODULO 5"
              # "Morphology Analysis"
              n307 = property on="Threshold Control" class="TabCtl (strict)"(error in=w365, "Visible"="1. Threshold") -> ()  [unwired: 1 in, 2 out]
              n308 = property on="Morphology Control" class="TabCtl (strict)"(error in=w365, "Visible"="2. Morphology") -> ()  [unwired: 1 in, 2 out]
              n309 = local read "Color Image"() -> (w364:T1)
              n310 = call "IMAQ Copy"("error in (no error)"=w365, "Image Dst"=w382, "Image Src"=w364) -> ("error out"=w384:errorcluster, "Image Dst Out"=w386:T1)  [unwired: 3 out]
              n311 = case shown="No Error" w384 {
                selector: w384 -> [w492 w555]
                tunnel: w386 -> [w498 w554]
                tunnel: w385 -> [w499 _]
                tunnel: w383 -> [w497 _]
                tunnel: w364 -> [w496 _]
                tunnel: [w494 w555] -> w380
                tunnel: [w493 w554] -> w379
                frame No Error {
                  n312 = case shown="\"Manual\"" "Threshold Control" {
                    tunnel: w498 -> [_ w548]
                    tunnel: w499 -> [w523 w547]
                    tunnel: [w522 w546] -> w493
                    tunnel: [w508 w544] -> w494
                    tunnel: w496 -> [w502 _]
                    tunnel: w497 -> [w504 _]
                    tunnel: w492 -> [w501 w536]
                    frame "Automatic", Default {
                      w518 = 2 items=["clustering", "entropy", "metric", "moments", "inter-class variance"] ("Method")
                      # "Umbraliza imagenes grises"
                      # "If Object Type is Dark AND the Method is metric, moment, or interclass variance, then invert the image."
                      # "The metric, moment, and interclass variance methods require doing the auto threshold on the inverse of the image when looking for dark objects."
                      n313 = call "IMAQ Copy"("error in (no error)"=w501, "Image Dst"=w504, "Image Src"=w502) -> ("error out"=w505:errorcluster, "Image Dst Out"=w503:T1)  [unwired: 3 out]
                      n314 = call "IMAQ ExtractSingleColorPlane"("Color Plane"="Color Plane", "error in (no error)"=w505, "Image Src"=w503) -> ("error out"=w506:errorcluster, "Image Dst Out"=w507:T1)  [unwired: 1 in, 6 out]
                      n315 = Unbundle By Name("Automatic") -> ("Object Type"=w520:u32, "Method"=w519:i32)
                      n316 = Not Equal To 0?(x=w520) -> (x != 0?=w511:bool)
                      n317 = Greater Or Equal?(x=w519, y=w518) -> (x >= y?=w510:bool)
                      n318 = And(x=w511, y=w510) -> (x .and. y?=w509:bool)
                      n319 = case shown="True" w509 {
                        tunnel: w507 -> [w524 w528]
                        tunnel: w523 -> [_ w529]
                        tunnel: [w524 w528] -> w513
                        tunnel: [w524 w527] -> w514
                        tunnel: [_ w526] -> w512
                        tunnel: w506 -> [_ w525]
                        frame False {
                        }
                        frame True {
                          n320 = call "IMAQ Inverse"("error in (no error)"=w525, "Image Dst"=w529, "Image Src"=w528) -> ("error out"=w526:errorcluster, "Image Dst Out"=w527:T1)  [unwired: 1 in, 6 out]
                        }
                      }
                      n321 = call "IMAQ AutoBThreshold"("error in (no error)"=w512, "Method"=w519, "Image"=w514) -> ("error out"=w517:errorcluster, "Threshold Value"=w515:i32)  [unwired: 1 in, 3 out]
                      "Threshold Value" <- w515
                      n322 = case shown="1" w520 {
                        tunnel: w515 -> [w531 w534]
                        tunnel: [w530 w533] -> w516
                        frame 0, Default {
                          # "Bright Objects"
                          n323 = Bundle("Threshold Value"=w531, 255) -> (w530:cluster{"Threshold Value":i32, i32})  [unwired: 1 out]
                        }
                        frame 1 {
                          # "Dark Objects"
                          n324 = Bundle(0, "Threshold Value"=w534) -> (w533:cluster{i32, "Threshold Value":i32})  [unwired: 1 out]
                        }
                      }
                      n325 = call "IMAQ Threshold"("error in (no error)"=w517, "Range"=w516, "Image Dst"=w523, "Image Src"=w513) -> ("error out"=w508:errorcluster, "Image Dst Out"=w522:T1)  [unwired: 2 in, 4 out]
                    }
                    frame "Manual" {
                      # "Dibuja histograma"
                      # "Convierte imagenes de color a binario a partir de un umbral"
                      n326 = local read "Histogram"() -> (w537:T7)
                      n327 = for {
                        tunnel: w537 -> [w549] mode=indexing
                        i -> [w550]
                        n328 = case shown="0, Default" w550 {
                          tunnel: w549 -> [w551 w552 w553]
                          frame 0, Default {
                            n329 = property on="Histogram Red" class="WFGraph (strict)"("Value"=w551) -> ()  [unwired: 2 in, 2 out]
                          }
                          frame 1 {
                            n330 = property on="Histogram Green" class="WFGraph (strict)"("Value"=w552) -> ()  [unwired: 2 in, 2 out]
                          }
                          frame 2 {
                            n331 = property on="Histogram Blue" class="WFGraph (strict)"("Value"=w553) -> ()  [unwired: 2 in, 2 out]
                          }
                        }
                      }
                      n332 = Unbundle("controls threshold") -> ("Threshold Color Mode"=w545:u16, "Color Value"=w543:i32, "Cluster Color"=w541:T39)
                      n333 = Unbundle(w541) -> ("Red or Hue Range"=w540:T40, "Green or Sat Range"=w539:T40, "Blue or Luma or Val or Inten Range"=w538:T40)  [unwired: 3 out]
                      n334 = call "IMAQ ColorThreshold"("Blue or Luma or Val or Inten Range"=w538, "Replace Value"=w543, "Green or Sat Range"=w539, "Color Mode"=w545, "error in (no error)"=w536, "Red or Hue Range"=w540, "Image Dst"=w547, "Image Src"=w548) -> ("error out"=w544:errorcluster, "Image Dst Out"=w546:T1)  [unwired: 2 out]
                    }
                  }
                }
                frame Error {
                }
              }
              n335 = call "IMAQ Copy"("error in (no error)"=w380, "Image Dst"=w378, "Image Src"=w379) -> ("error out"=w363:errorcluster, "Image Dst Out"=w373:T1)  [unwired: 3 out]
              "Threshold Image" <- w373
              n336 = call "IMAQ Copy"("error in (no error)"=w363, "Image Dst"=w371, "Image Src"=w373) -> ("error out"=w375:errorcluster, "Image Dst Out"=w374:T1)  [unwired: 3 out]
              n337 = property on="Particle Connectivity Control" class="Bool (strict)"("Visible"="4. Particle Connectivity") -> ()  [unwired: 2 in, 2 out]
              n338 = stacked-sequence {
                seq-local: [w404 _ _ _ _] -> [_ w426 _ _ _]
                seq-local: [w405 _ _ _ _] -> [_ w423 _ _ _]
                seq-local: [_ w427 _ _ _] -> [_ _ w444 _ _]
                seq-local: [_ w425 _ _ _] -> [_ _ w442 _ _]
                seq-local: [_ _ w443 _ _] -> [_ _ _ w461 _]
                seq-local: [_ _ w441 _ _] -> [_ _ _ w460 _]
                seq-local: [_ _ _ w455 _] -> [_ _ _ _ w478]
                seq-local: [_ _ _ w456 _] -> [_ _ _ _ w476]
                tunnel: w374 -> [w409 _ _ _ _]
                tunnel: w370 -> [w403 w424 w440 w457 w477]
                tunnel: w375 -> [w408 _ _ _ _]
                tunnel: [_ _ _ _ w475] -> w377
                tunnel: [_ _ _ _ w474] -> w376
                frame #0 {
                  # "Remueve particulas pequeñas"
                  n339 = Not Equal To 0?(x="Particles to Erode") -> (x != 0?=w406:bool)
                  n340 = case shown="True" w406 {
                    tunnel: w409 -> [w411 w414]
                    tunnel: w408 -> [w410 w413]
                    tunnel: "Particles to Erode" -> [_ w419]
                    tunnel: [w410 w418] -> w405
                    tunnel: [w411 w417] -> w404
                    tunnel: w403 -> [_ w412]
                    frame False {
                    }
                    frame True {
                      n341 = call "IMAQ Copy"("error in (no error)"=w413, "Image Dst"=w412, "Image Src"=w414) -> ("error out"=w416:errorcluster, "Image Dst Out"=w415:T1)  [unwired: 3 out]
                      n342 = call "IMAQ RemoveParticle"("Connectivity 4/8 (8)"="Connectivity for Particle Erosion", "Low Pass/High Pass (Low)"="Filter", "Square/Hexa (Square)"="Neighborhood", "error in (no error)"=w416, "Number of Erosion"=w419, "Image Src"=w415) -> ("error out"=w418:errorcluster, "Image Dst Out"=w417:T1)  [unwired: 1 in, 3 out]
                    }
                  }
                }
                frame #1 {
                  # "Remueve particulas en el borde"
                  n343 = case shown="False" "Reject Particles Touching the Image Border" {
                    tunnel: [w429 w437] -> w427
                    tunnel: w426 -> [w430 w433]
                    tunnel: [w430 w436] -> w425
                    tunnel: w424 -> [_ w432]
                    tunnel: w423 -> [w429 w431]
                    frame False {
                    }
                    frame True {
                      n344 = call "IMAQ Copy"("error in (no error)"=w431, "Image Dst"=w432, "Image Src"=w433) -> ("error out"=w435:errorcluster, "Image Dst Out"=w434:T1)  [unwired: 3 out]
                      n345 = call "IMAQ RejectBorder"("error in (no error)"=w435, "Image Src"=w434, "Connectivity 4/8 (8)"="Connectivity for Border Rejection") -> ("error out"=w437:errorcluster, "Image Dst Out"=w436:T1)  [unwired: 1 in, 2 out]
                    }
                  }
                }
                frame #2 {
                  # "Rellena agujeros"
                  n346 = case shown="False" "Fill Holes" {
                    tunnel: w444 -> [w445 w451]
                    tunnel: [w445 w453] -> w443
                    tunnel: w442 -> [w446 w449]
                    tunnel: [w446 w452] -> w441
                    tunnel: w440 -> [_ w448]
                    frame False {
                    }
                    frame True {
                      n347 = call "IMAQ Copy"("error in (no error)"=w451, "Image Dst"=w448, "Image Src"=w449) -> ("error out"=w450:errorcluster, "Image Dst Out"=w447:T1)  [unwired: 3 out]
                      n348 = call "IMAQ FillHole"("error in (no error)"=w450, "Image Src"=w447, "Connectivity 4/8 (8)"="Connectivity for Hole Filling") -> ("error out"=w453:errorcluster, "Image Dst Out"=w452:T1)  [unwired: 1 in, 2 out]
                    }
                  }
                }
                frame #3 {
                  # "Separa particulas"
                  n349 = Not Equal To 0?(x="Separation Erosion") -> (x != 0?=w459:bool)
                  n350 = case shown="True" w459 {
                    tunnel: w461 -> [w462 w467]
                    tunnel: w460 -> [w463 w465]
                    tunnel: "Separation Erosion" -> [_ w472]
                    tunnel: w457 -> [_ w466]
                    tunnel: [w462 w470] -> w456
                    tunnel: [w463 w469] -> w455
                    frame False {
                    }
                    frame True {
                      n351 = call "IMAQ Copy"("error in (no error)"=w467, "Image Dst"=w466, "Image Src"=w465) -> ("error out"=w468:errorcluster, "Image Dst Out"=w464:T1)  [unwired: 3 out]
                      n352 = call "IMAQ Separation"("Square/Hexa (Square)"="Morphology for Separation Erosion", "error in (no error)"=w468, "Nb of Erosion"=w472, "Image Src"=w464) -> ("error out"=w470:errorcluster, "Image Dst Out"=w469:T1)  [unwired: 2 in, 4 out]
                    }
                  }
                }
                frame #4 {
                  # "Conserva/elimina particulas segun criterio"
                  n353 = case shown="True" "Particle Filter" {
                    tunnel: w478 -> [w480 w483]
                    tunnel: w477 -> [_ w482]
                    tunnel: w476 -> [w479 w481]
                    tunnel: [w479 w491] -> w475
                    tunnel: [w480 w490] -> w474
                    frame False {
                    }
                    frame True {
                      n354 = call "IMAQ Copy"("error in (no error)"=w481, "Image Dst"=w482, "Image Src"=w483) -> ("error out"=w484:errorcluster, "Image Dst Out"=w485:T1)  [unwired: 3 out]
                      n355 = call "IMAQ Particle Filter 2"("Keep/Remove Particles (F)"="Keep/Remove PF", "Connectivity 4/8 (8)"="Connectivity for PF", "error in (no error)"=w484, "Selection Values"="Particle Filter Values", "Image Src"=w485) -> ("error out"=w491:errorcluster, "Number of Particles"=→"Particles":i32, "Image Dst Out"=w490:T1)  [unwired: 3 in, 1 out]
                    }
                  }
                }
              }
              n356 = call "IMAQ Copy"("error in (no error)"=w377, "Image Dst"=w372, "Image Src"=w376) -> ("error out"=w362:errorcluster, "Image Dst Out"=w368:T1)  [unwired: 3 out]
              "Morphology Image" <- w368
              n357 = case shown="True" "4. Particle Connectivity" {
                tunnel: w369 -> [_ w393]
                tunnel: w362 -> [w387 w392]
                tunnel: w368 -> [_ w391]
                tunnel: [w387 w390] -> w361
                tunnel: [_ w389] -> w360
                tunnel: [_ w388] -> w359
                frame False {
                }
                frame True {
                  n358 = call "IMAQ Copy"("error in (no error)"=w392, "Image Dst"=w393, "Image Src"=w391) -> ("error out"=w394:errorcluster, "Image Dst Out"=w395:T1)  [unwired: 3 out]
                  n359 = case shown="No Error" w394 {
                    selector: w394 -> [w401 w402]
                    tunnel: [w398 w402] -> w390
                    tunnel: w395 -> [w399 _]
                    tunnel: [w397 _] -> w389
                    tunnel: [w396 _] -> w388
                    frame No Error {
                      # "Analiza todas las particulas que halla"
                      n360 = call "IMAQ Particle Analysis Report"("Connectivity 4/8 (8)"="Particle Connectivity Control", "error in (no error)"=w401, "Image"=w399) -> ("error out"=w398:errorcluster, "Particle Reports (Pixels)"=w396:T29, "Number of Particles"=w397:i32)  [unwired: 6 out]
                    }
                    frame Error {
                    }
                  }
                }
              }
              n361 = Bundle("Particle Reports (Pixels)"=w359, "Number of Particles"=w360) -> (→"Cluster Particle Reports (Pixels) Out":T41)  [unwired: 1 out]
            }
          }
        }
        n362 = case shown="True" TRUE {
          tunnel: [errorcluster {"status"=FALSE, "code"=0, "source"=""} ("error IO") w662] -> w235
          tunnel: w211 -> [_ w660]
          tunnel: w210 -> [_ w659]
          tunnel: w209 -> [_ w658]
          frame False {
          }
          frame True {
            n363 = for {
              N: 1 -> [_]
              tunnel: w660 -> [w676]
              tunnel: w658 -> [w675]
              tunnel: [w663] -> w662
              tunnel: w659 -> [w664]
              # "MODULO 6"
              n364 = local read "Morphology Image"() -> (w665:T1)
              n365 = local read "Numeric Tab control"() -> (w666:i32)
              n366 = case shown="1" w666 {
                tunnel: [_ w677] -> w667
                frame 0, Default {
                }
                frame 1 {
                  n367 = property on="Result Picture" class="Pict"() -> ("Mouse"=w677:T34)  [unwired: 2 in, 2 out]
                }
              }
              n368 = Unbundle(w667) -> ("Mouse Position"=w670:cluster{"X":i32, "Y":i32}, "Mouse Modifiers"=w673:T42)
              n369 = Unbundle By Name(w673) -> ("Button Down"=w672:bool)
              n370 = Cluster To Array(cluster=w670) -> (array=w671:i32[])
              n371 = call "IMAQ Copy"("error in (no error)"=w664, "Image Dst"=w675, "Image Src"=w665) -> ("error out"=w668:errorcluster, "Image Dst Out"=w669:T1)  [unwired: 3 out]
              n372 = property on="Shape Control" class="Clust (strict)"(error in=w664, "Visible"="3. Shape") -> ()  [unwired: 1 in, 2 out]
              n373 = case shown="No Error" w668 {
                selector: w668 -> [w685 w719]
                tunnel: w671 -> [w687 _]
                tunnel: w676 -> [w690 _]
                tunnel: w669 -> [w683 _]
                tunnel: w672 -> [w689 _]
                tunnel: [w684 w719] -> w663
                frame No Error {
                  # "When the user clicks on the image, we index the image \nto get the value of the pixel that was clicked on. \nThis color is used to mask the image."
                  # "Hay Template?"
                  n374 = case shown="True" w689 {
                    tunnel: [w708 w715] -> w681
                    tunnel: w687 -> [_ w714]
                    tunnel: w690 -> [_ w713]
                    tunnel: [w709 w711] -> w678
                    tunnel: w683 -> [_ w712]
                    tunnel: w685 -> [w708 w710]
                    frame False {
                      n375 = local read "MagicWand Image"() -> (w709:T1)
                    }
                    frame True {
                      # "Select entire object"
                      n376 = call "IMAQ MagicWand"("Connectivity 4/8 (8)"=TRUE, "Tolerance"=sgl 0.0, "Fill Value"=u8 1, "error in (no error)"=w710, "Hot spot (x,y)"=w714, "Image Dst"=w713, "Image Src"=w712) -> ("error out"=w715:errorcluster, "Image Dst Out"=w711:T1)  [unwired: 3 out]
                      "MagicWand Image" <- w711
                    }
                  }
                  n377 = Unbundle By Name("Shape Control") -> ("Scale Invariance"=w693:bool, "Tolerance (%)"=w692:dbl, "Connectivity"=w691:bool)
                  n378 = Unbundle(w678) -> (w680:string)  [unwired: 1 out]
                  n379 = Empty String/Path?(string/path=w680) -> (empty?=w679:bool)
                  n380 = Divide(x=w692, y=100) -> (x/y=w696:dbl)
                  n381 = case shown="False" w679 {
                    tunnel: w696 -> [w705 _]
                    tunnel: w693 -> [w704 _]
                    tunnel: w691 -> [w703 _]
                    tunnel: [w700 w706] -> w684
                    tunnel: w681 -> [w702 w707]
                    tunnel: w683 -> [w701 _]
                    tunnel: [w699 _] -> w688
                    tunnel: [w698 _] -> w686
                    tunnel: w678 -> [w697 _]
                    frame False {
                      n382 = call "IMAQ Shape Match Tool"("Scale Invariance? (Yes)"=w704, "Connectivity 4/8 (8)"=w703, "Tolerance"=w705, "error in (no error)"=w702, "Image Template"=w697, "Image Src"=w701) -> ("error out"=w700:errorcluster, "Shape Report"=w699:T30, "Number of Matches"=w698:i32)  [unwired: 1 in, 2 out]
                    }
                    frame True {
                      # "Elimina error cuando\nno se ha echo ninguna\nprimera busqueda."
                      n383 = call "Clear Errors.vi"("error in (no error)"=w707) -> ("error out"=w706:errorcluster)  [unwired: 6 out]
                    }
                  }
                  n384 = Bundle("Shape Report"=w688, "Number of Matches"=w686) -> (→"Cluster Shape Report Out":T43)  [unwired: 1 out]
                }
                frame Error {
                }
              }
            }
          }
        }
        n385 = local read "stop 2"() -> (w232:bool)
      }
    }
    frame #2 {
      w1092 = FALSE
      # "Copyright 2008 PACW"
      # "Finalización de botones"
      # "Libera espacio\nde memoria de\nimagen."
      n386 = Merge Errors(w1095, w1096) -> (w1097:errorcluster)
      n387 = case shown="False" w1086 {
        tunnel: w1089 -> [w1107 w1108]
        tunnel: [w1106 w1108] -> w1088
        tunnel: w1087 -> [w1105 _]
        frame False {
          n388 = call <vilib>:"IMAQdx Close Camera.vi"("error in"=w1107, "Session In"=w1105) -> ("error out"=w1106:errorcluster)  [unwired: 9 in]
        }
        frame True {
        }
      }
      n389 = Merge Errors(w1094, w1093, w1097) -> (w1100:errorcluster)
      n390 = Merge Errors(w1091, w1101, w1100) -> (w1102:errorcluster)
      n391 = call "IMAQ Dispose"("All Images? (No)"=TRUE, "Image"=w1098, "error in (no error)"=w1088) -> ("error out"=w1099:errorcluster)  [unwired: 3 out]
      n392 = local write "stop 2"(w1092) -> ()
      n393 = local write "Acquiring"(w1092) -> ()
      n394 = local write "stop"(w1092) -> ()
      n395 = local write "Play"(w1092) -> ()
      n396 = local write "Pause"(w1092) -> ()
      n397 = local write "Subtraction"(w1092) -> ()
      n398 = Merge Errors(w1099, w1090, w1102) -> (w1103:errorcluster)
      n399 = call "Simple Error Handler.vi"("error in (no error)"=w1103) -> ()  [unwired: 1 in, 8 out]
    }
  }
